vi "MultirunBuilderForNamedLocations2.vi"() -> ()   [LabVIEW 2015]
uses:
  Anemometry Sub Vis/Gen Trav/Spacing.ctl
  Anemometry Sub Vis/Controls/Multi_run_mode.ctl
  MultirunBuilderSubVIs/MRBRowTaskSelector.ctl
  Anemometry Sub Vis/File/Setup_Filetype.ctl
  Anemometry Sub Vis/Controls/Tunnel_Coordinates.ctl
  Anemometry Sub Vis/Globals/Meas_global.vi
  MultirunBuilderSubVIs/MRCMDFBGlobal.vi
  MultirunBuilderSubVIs/Set Speed Only.vi
  MultirunBuilderSubVIs/Wait (minutes).vi
  MultirunBuilderSubVIs/Single Measurement.vi
  MultirunBuilderSubVIs/Auto Calibrate.vi
  MultirunBuilderSubVIs/MoveTT.vi
panel:
  in  "Vert.Z-Locations 2":dbl[](array[numeric])=[12.7, 19.05, 25.4]
  in  "TaskArray":T3(array[cluster])=[{"Start X"=-3390.0, "Start Y"=-113.0, "Start Z"=780.0, "End X"=-3390.0, "End Y"=-113.0, "End Z"=780.0, "No. of pts."=0, "Spacing"=enum."Linear", "Filename"=path "", "Tunnel Speed"=7.64, "Averaging time (min)"=0.0, "Extra Commands"="", "Carrier_1 Q (l/min)"=0.0, "Carrier_2 Q (l/min)"=0.0, "Trace Gas Concentration (%)"=0.0, "Specific Arguments"="", "Comments"="Tunnel Warm Up", "Row No"=0, "Row Type Selector"=enum."Set Tunnel Speed Only", "Completion time"="", "Row Duration (mins)"=10.0, "No. of Valid pts."=0, "Meas Setup File"=""}, {"Start X"=-3390.0, "Start Y"=-113.0, "Start Z"=780.0, "End X"=-3390.0, "End Y"=-113.0, "End Z"=780.0, "No. of pts."=0, "Spacing"=enum."Linear", "Filename"=path "", "Tunnel Speed"=7.64, "Averaging time (min)"=0.0, "Extra Commands"="", "Carrier_1 Q (l/min)"=0.0, "Carrier_2 Q (l/min)"=0.0, "Trace Gas Concentration (%)"=0.0, "Specific Arguments"="10", "Comments"="Tunnel Warm Up", "Row No"=0, "Row Type Selector"=enum."Wait (minutes)", "Completion time"="", "Row Duration (mins)"=0.0, "No. of Valid pts."=0, "Meas Setup File"=""}, {"Start X"=0.0, "Start Y"=0.0, "Start Z"=150.0, "End X"=0.0, "End Y"=0.0, "End Z"=150.0, "No. of pts."=0, "Spacing"=enum."Linear", "Filename"=path "", "Tunnel Speed"=7.64, "Averaging time (min)"=0.0, "Extra Commands"="!Work in Tunnel Coordinates", "Carrier_1 Q (l/min)"=0.0, "Carrier_2 Q (l/min)"=0.0, "Trace Gas Concentration (%)"=0.0, "Specific Arguments"="", "Comments"="", "Row No"=0, "Row Type Selector"=enum."Move Traverse Only", "Completion time"="", "Row Duration (mins)"=0.0, "No. of Valid pts."=0, "Meas Setup File"=""}, {"Start X"=0.0, "Start Y"=0.0, "Start Z"=805.0, "End X"=0.0, "End Y"=0.0, "End Z"=805.0, "No. of pts."=0, "Spacing"=enum."Linear", "Filename"=path "", "Tunnel Speed"=7.64, "Averaging time (min)"=0.0, "Extra Commands"="!Work in Tunnel Coordinates", "Carrier_1 Q (l/min)"=0.0, "Carrier_2 Q (l/min)"=0.0, "Trace Gas Concentration (%)"=0.0, "Specific Arguments"="MoveTT.vi;10", "Comments"="", "Row No"=0, "Row Type Selector"=enum."Run VI Named:", "Completion time"="", "Row Duration (mins)"=0.0, "No. of Valid pts."=0, "Meas Setup File"=""}, {"Start X"=-72.9, "Start Y"=-56.5, "Start Z"=12.7, "End X"=-72.9, "End Y"=-56.5, "End Z"=25.4, "No. of pts."=3, "Spacing"=enum."Specified", "Filename"=path "M:/\\Projects\\8773\\Results\\Tunnel1\\AnemometerSurvey.xls", "Tunnel Speed"=7.64, "Averaging time (min)"=1.0, "Extra Commands"="", "Carrier_1 Q (l/min)"=0.0, "Carrier_2 Q (l/min)"=0.0, "Trace Gas Concentration (%)"=0.0, "Specific Arguments"="Z= ;12.7;19.1;25.4\r", "Comments"="Anemo1", "Row No"=0, "Row Type Selector"=enum."Vertical Profile", "Completion time"="", "Row Duration (mins)"=0.0, "No. of Valid pts."=0, "Meas Setup File"="Current_Setup.xls"}, {"Start X"=-458.4, "Start Y"=87.9, "Start Z"=25.6, "End X"=-458.4, "End Y"=87.9, "End Z"=38.3, "No. of pts."=3, "Spacing"=enum."Specified", "Filename"=path "M:/\\Projects\\8773\\Results\\Tunnel1\\AnemometerSurvey.xls", "Tunnel Speed"=7.64, "Averaging time (min)"=1.0, "Extra Commands"="", "Carrier_1 Q (l/min)"=0.0, "Carrier_2 Q (l/min)"=0.0, "Trace Gas Concentration (%)"=0.0, "Specific Arguments"="Z= ;25.6;32.0;38.3\r", "Comments"="Anemo2", "Row No"=0, "Row Type Selector"=enum."Vertical Profile", "Completion time"="", "Row Duration (mins)"=0.0, "No. of Valid pts."=0, "Meas Setup File"="Current_Setup.xls"}, {"Start X"=0.0, "Start Y"=0.0, "Start Z"=150.0, "End X"=0.0, "End Y"=0.0, "End Z"=150.0, "No. of pts."=0, "Spacing"=enum."Linear", "Filename"=path "", "Tunnel Speed"=7.64, "Averaging time (min)"=0.0, "Extra Commands"="!Work in Tunnel Coordinates", "Carrier_1 Q (l/min)"=0.0, "Carrier_2 Q (l/min)"=0.0, "Trace Gas Concentration (%)"=0.0, "Specific Arguments"="", "Comments"="", "Row No"=0, "Row Type Selector"=enum."Move Traverse Only", "Completion time"="", "Row Duration (mins)"=0.0, "No. of Valid pts."=0, "Meas Setup File"=""}, {"Start X"=0.0, "Start Y"=0.0, "Start Z"=805.0, "End X"=0.0, "End Y"=0.0, "End Z"=805.0, "No. of pts."=0, "Spacing"=enum."Linear", "Filename"=path "", "Tunnel Speed"=7.64, "Averaging time (min)"=0.0, "Extra Commands"="!Work in Tunnel Coordinates", "Carrier_1 Q (l/min)"=0.0, "Carrier_2 Q (l/min)"=0.0, "Trace Gas Concentration (%)"=0.0, "Specific Arguments"="MoveTT.vi;30", "Comments"="", "Row No"=0, "Row Type Selector"=enum."Run VI Named:", "Completion time"="", "Row Duration (mins)"=0.0, "No. of Valid pts."=0, "Meas Setup File"=""}, {"Start X"=-72.9, "Start Y"=-56.5, "Start Z"=12.7, "End X"=-72.9, "End Y"=-56.5, "End Z"=25.4, "No. of pts."=3, "Spacing"=enum."Specified", "Filename"=path "M:/\\Projects\\8773\\Results\\Tunnel1\\AnemometerSurvey.xls", "Tunnel Speed"=7.64, "Averaging time (min)"=1.0, "Extra Commands"="", "Carrier_1 Q (l/min)"=0.0, "Carrier_2 Q (l/min)"=0.0, "Trace Gas Concentration (%)"=0.0, "Specific Arguments"="Z= ;12.7;19.1;25.4\r", "Comments"="Anemo1", "Row No"=0, "Row Type Selector"=enum."Vertical Profile", "Completion time"="", "Row Duration (mins)"=0.0, "No. of Valid pts."=0, "Meas Setup File"="Current_Setup.xls"}, {"Start X"=-458.4, "Start Y"=87.9, "Start Z"=25.6, "End X"=-458.4, "End Y"=87.9, "End Z"=38.3, "No. of pts."=3, "Spacing"=enum."Specified", "Filename"=path "M:/\\Projects\\8773\\Results\\Tunnel1\\AnemometerSurvey.xls", "Tunnel Speed"=7.64, "Averaging time (min)"=1.0, "Extra Commands"="", "Carrier_1 Q (l/min)"=0.0, "Carrier_2 Q (l/min)"=0.0, "Trace Gas Concentration (%)"=0.0, "Specific Arguments"="Z= ;25.6;32.0;38.3\r", "Comments"="Anemo2", "Row No"=0, "Row Type Selector"=enum."Vertical Profile", "Completion time"="", "Row Duration (mins)"=0.0, "No. of Valid pts."=0, "Meas Setup File"="Current_Setup.xls"}, {"Start X"=0.0, "Start Y"=0.0, "Start Z"=150.0, "End X"=0.0, "End Y"=0.0, "End Z"=150.0, "No. of pts."=0, "Spacing"=enum."Linear", "Filename"=path "", "Tunnel Speed"=7.64, "Averaging time (min)"=0.0, "Extra Commands"="!Work in Tunnel Coordinates", "Carrier_1 Q (l/min)"=0.0, "Carrier_2 Q (l/min)"=0.0, "Trace Gas Concentration (%)"=0.0, "Specific Arguments"="", "Comments"="", "Row No"=0, "Row Type Selector"=enum."Move Traverse Only", "Completion time"="", "Row Duration (mins)"=0.0, "No. of Valid pts."=0, "Meas Setup File"=""}, {"Start X"=0.0, "Start Y"=0.0, "Start Z"=805.0, "End X"=0.0, "End Y"=0.0, "End Z"=805.0, "No. of pts."=0, "Spacing"=enum."Linear", "Filename"=path "", "Tunnel Speed"=7.64, "Averaging time (min)"=0.0, "Extra Commands"="!Work in Tunnel Coordinates", "Carrier_1 Q (l/min)"=0.0, "Carrier_2 Q (l/min)"=0.0, "Trace Gas Concentration (%)"=0.0, "Specific Arguments"="MoveTT.vi;50", "Comments"="", "Row No"=0, "Row Type Selector"=enum."Run VI Named:", "Completion time"="", "Row Duration (mins)"=0.0, "No. of Valid pts."=0, "Meas Setup File"=""}, {"Start X"=-72.9, "Start Y"=-56.5, "Start Z"=12.7, "End X"=-72.9, "End Y"=-56.5, "End Z"=25.4, "No. of pts."=3, "Spacing"=enum."Specified", "Filename"=path "M:/\\Projects\\8773\\Results\\Tunnel1\\AnemometerSurvey.xls", "Tunnel Speed"=7.64, "Averaging time (min)"=1.0, "Extra Commands"="", "Carrier_1 Q (l/min)"=0.0, "Carrier_2 Q (l/min)"=0.0, "Trace Gas Concentration (%)"=0.0, "Specific Arguments"="Z= ;12.7;19.1;25.4\r", "Comments"="Anemo1", "Row No"=0, "Row Type Selector"=enum."Vertical Profile", "Completion time"="", "Row Duration (mins)"=0.0, "No. of Valid pts."=0, "Meas Setup File"="Current_Setup.xls"}, {"Start X"=-458.4, "Start Y"=87.9, "Start Z"=25.6, "End X"=-458.4, "End Y"=87.9, "End Z"=38.3, "No. of pts."=3, "Spacing"=enum."Specified", "Filename"=path "M:/\\Projects\\8773\\Results\\Tunnel1\\AnemometerSurvey.xls", "Tunnel Speed"=7.64, "Averaging time (min)"=1.0, "Extra Commands"="", "Carrier_1 Q (l/min)"=0.0, "Carrier_2 Q (l/min)"=0.0, "Trace Gas Concentration (%)"=0.0, "Specific Arguments"="Z= ;25.6;32.0;38.3\r", "Comments"="Anemo2", "Row No"=0, "Row Type Selector"=enum."Vertical Profile", "Completion time"="", "Row Duration (mins)"=0.0, "No. of Valid pts."=0, "Meas Setup File"="Current_Setup.xls"}, {"Start X"=0.0, "Start Y"=0.0, "Start Z"=150.0, "End X"=0.0, "End Y"=0.0, "End Z"=150.0, "No. of pts."=0, "Spacing"=enum."Linear", "Filename"=path "", "Tunnel Speed"=7.64, "Averaging time (min)"=0.0, "Extra Commands"="!Work in Tunnel Coordinates", "Carrier_1 Q (l/min)"=0.0, "Carrier_2 Q (l/min)"=0.0, "Trace Gas Concentration (%)"=0.0, "Specific Arguments"="", "Comments"="", "Row No"=0, "Row Type Selector"=enum."Move Traverse Only", "Completion time"="", "Row Duration (mins)"=0.0, "No. of Valid pts."=0, "Meas Setup File"=""}, {"Start X"=0.0, "Start Y"=0.0, "Start Z"=805.0, "End X"=0.0, "End Y"=0.0, "End Z"=805.0, "No. of pts."=0, "Spacing"=enum."Linear", "Filename"=path "", "Tunnel Speed"=7.64, "Averaging time (min)"=0.0, "Extra Commands"="!Work in Tunnel Coordinates", "Carrier_1 Q (l/min)"=0.0, "Carrier_2 Q (l/min)"=0.0, "Trace Gas Concentration (%)"=0.0, "Specific Arguments"="MoveTT.vi;70", "Comments"="", "Row No"=0, "Row Type Selector"=enum."Run VI Named:", "Completion time"="", "Row Duration (mins)"=0.0, "No. of Valid pts."=0, "Meas Setup File"=""}, {"Start X"=-72.9, "Start Y"=-56.5, "Start Z"=12.7, "End X"=-72.9, "End Y"=-56.5, "End Z"=25.4, "No. of pts."=3, "Spacing"=enum."Specified", "Filename"=path "M:/\\Projects\\8773\\Results\\Tunnel1\\AnemometerSurvey.xls", "Tunnel Speed"=7.64, "Averaging time (min)"=1.0, "Extra Commands"="", "Carrier_1 Q (l/min)"=0.0, "Carrier_2 Q (l/min)"=0.0, "Trace Gas Concentration (%)"=0.0, "Specific Arguments"="Z= ;12.7;19.1;25.4\r", "Comments"="Anemo1", "Row No"=0, "Row Type Selector"=enum."Vertical Profile", "Completion time"="", "Row Duration (mins)"=0.0, "No. of Valid pts."=0, "Meas Setup File"="Current_Setup.xls"}, {"Start X"=-458.4, "Start Y"=87.9, "Start Z"=25.6, "End X"=-458.4, "End Y"=87.9, "End Z"=38.3, "No. of pts."=3, "Spacing"=enum."Specified", "Filename"=path "M:/\\Projects\\8773\\Results\\Tunnel1\\AnemometerSurvey.xls", "Tunnel Speed"=7.64, "Averaging time (min)"=1.0, "Extra Commands"="", "Carrier_1 Q (l/min)"=0.0, "Carrier_2 Q (l/min)"=0.0, "Trace Gas Concentration (%)"=0.0, "Specific Arguments"="Z= ;25.6;32.0;38.3\r", "Comments"="Anemo2", "Row No"=0, "Row Type Selector"=enum."Vertical Profile", "Completion time"="", "Row Duration (mins)"=0.0, "No. of Valid pts."=0, "Meas Setup File"="Current_Setup.xls"}, {"Start X"=0.0, "Start Y"=0.0, "Start Z"=150.0, "End X"=0.0, "End Y"=0.0, "End Z"=150.0, "No. of pts."=0, "Spacing"=enum."Linear", "Filename"=path "", "Tunnel Speed"=7.64, "Averaging time (min)"=0.0, "Extra Commands"="!Work in Tunnel Coordinates", "Carrier_1 Q (l/min)"=0.0, "Carrier_2 Q (l/min)"=0.0, "Trace Gas Concentration (%)"=0.0, "Specific Arguments"="", "Comments"="", "Row No"=0, "Row Type Selector"=enum."Move Traverse Only", "Completion time"="", "Row Duration (mins)"=0.0, "No. of Valid pts."=0, "Meas Setup File"=""}, {"Start X"=0.0, "Start Y"=0.0, "Start Z"=805.0, "End X"=0.0, "End Y"=0.0, "End Z"=805.0, "No. of pts."=0, "Spacing"=enum."Linear", "Filename"=path "", "Tunnel Speed"=7.64, "Averaging time (min)"=0.0, "Extra Commands"="!Work in Tunnel Coordinates", "Carrier_1 Q (l/min)"=0.0, "Carrier_2 Q (l/min)"=0.0, "Trace Gas Concentration (%)"=0.0, "Specific Arguments"="MoveTT.vi;90", "Comments"="", "Row No"=0, "Row Type Selector"=enum."Run VI Named:", "Completion time"="", "Row Duration (mins)"=0.0, "No. of Valid pts."=0, "Meas Setup File"=""}, {"Start X"=-72.9, "Start Y"=-56.5, "Start Z"=12.7, "End X"=-72.9, "End Y"=-56.5, "End Z"=25.4, "No. of pts."=3, "Spacing"=enum."Specified", "Filename"=path "M:/\\Projects\\8773\\Results\\Tunnel1\\AnemometerSurvey.xls", "Tunnel Speed"=7.64, "Averaging time (min)"=1.0, "Extra Commands"="", "Carrier_1 Q (l/min)"=0.0, "Carrier_2 Q (l/min)"=0.0, "Trace Gas Concentration (%)"=0.0, "Specific Arguments"="Z= ;12.7;19.1;25.4\r", "Comments"="Anemo1", "Row No"=0, "Row Type Selector"=enum."Vertical Profile", "Completion time"="", "Row Duration (mins)"=0.0, "No. of Valid pts."=0, "Meas Setup File"="Current_Setup.xls"}, {"Start X"=-458.4, "Start Y"=87.9, "Start Z"=25.6, "End X"=-458.4, "End Y"=87.9, "End Z"=38.3, "No. of pts."=3, "Spacing"=enum."Specified", "Filename"=path "M:/\\Projects\\8773\\Results\\Tunnel1\\AnemometerSurvey.xls", "Tunnel Speed"=7.64, "Averaging time (min)"=1.0, "Extra Commands"="", "Carrier_1 Q (l/min)"=0.0, "Carrier_2 Q (l/min)"=0.0, "Trace Gas Concentration (%)"=0.0, "Specific Arguments"="Z= ;25.6;32.0;38.3\r", "Comments"="Anemo2", "Row No"=0, "Row Type Selector"=enum."Vertical Profile", "Completion time"="", "Row Duration (mins)"=0.0, "No. of Valid pts."=0, "Meas Setup File"="Current_Setup.xls"}, {"Start X"=0.0, "Start Y"=0.0, "Start Z"=150.0, "End X"=0.0, "End Y"=0.0, "End Z"=150.0, "No. of pts."=0, "Spacing"=enum."Linear", "Filename"=path "", "Tunnel Speed"=7.64, "Averaging time (min)"=0.0, "Extra Commands"="!Work in Tunnel Coordinates", "Carrier_1 Q (l/min)"=0.0, "Carrier_2 Q (l/min)"=0.0, "Trace Gas Concentration (%)"=0.0, "Specific Arguments"="", "Comments"="", "Row No"=0, "Row Type Selector"=enum."Move Traverse Only", "Completion time"="", "Row Duration (mins)"=0.0, "No. of Valid pts."=0, "Meas Setup File"=""}, {"Start X"=0.0, "Start Y"=0.0, "Start Z"=805.0, "End X"=0.0, "End Y"=0.0, "End Z"=805.0, "No. of pts."=0, "Spacing"=enum."Linear", "Filename"=path "", "Tunnel Speed"=7.64, "Averaging time (min)"=0.0, "Extra Commands"="!Work in Tunnel Coordinates", "Carrier_1 Q (l/min)"=0.0, "Carrier_2 Q (l/min)"=0.0, "Trace Gas Concentration (%)"=0.0, "Specific Arguments"="MoveTT.vi;110", "Comments"="", "Row No"=0, "Row Type Selector"=enum."Run VI Named:", "Completion time"="", "Row Duration (mins)"=0.0, "No. of Valid pts."=0, "Meas Setup File"=""}, {"Start X"=-72.9, "Start Y"=-56.5, "Start Z"=12.7, "End X"=-72.9, "End Y"=-56.5, "End Z"=25.4, "No. of pts."=3, "Spacing"=enum."Specified", "Filename"=path "M:/\\Projects\\8773\\Results\\Tunnel1\\AnemometerSurvey.xls", "Tunnel Speed"=7.64, "Averaging time (min)"=1.0, "Extra Commands"="", "Carrier_1 Q (l/min)"=0.0, "Carrier_2 Q (l/min)"=0.0, "Trace Gas Concentration (%)"=0.0, "Specific Arguments"="Z= ;12.7;19.1;25.4\r", "Comments"="Anemo1", "Row No"=0, "Row Type Selector"=enum."Vertical Profile", "Completion time"="", "Row Duration (mins)"=0.0, "No. of Valid pts."=0, "Meas Setup File"="Current_Setup.xls"}, {"Start X"=-458.4, "Start Y"=87.9, "Start Z"=25.6, "End X"=-458.4, "End Y"=87.9, "End Z"=38.3, "No. of pts."=3, "Spacing"=enum."Specified", "Filename"=path "M:/\\Projects\\8773\\Results\\Tunnel1\\AnemometerSurvey.xls", "Tunnel Speed"=7.64, "Averaging time (min)"=1.0, "Extra Commands"="", "Carrier_1 Q (l/min)"=0.0, "Carrier_2 Q (l/min)"=0.0, "Trace Gas Concentration (%)"=0.0, "Specific Arguments"="Z= ;25.6;32.0;38.3\r", "Comments"="Anemo2", "Row No"=0, "Row Type Selector"=enum."Vertical Profile", "Completion time"="", "Row Duration (mins)"=0.0, "No. of Valid pts."=0, "Meas Setup File"="Current_Setup.xls"}, {"Start X"=0.0, "Start Y"=0.0, "Start Z"=150.0, "End X"=0.0, "End Y"=0.0, "End Z"=150.0, "No. of pts."=0, "Spacing"=enum."Linear", "Filename"=path "", "Tunnel Speed"=7.64, "Averaging time (min)"=0.0, "Extra Commands"="!Work in Tunnel Coordinates", "Carrier_1 Q (l/min)"=0.0, "Carrier_2 Q (l/min)"=0.0, "Trace Gas Concentration (%)"=0.0, "Specific Arguments"="", "Comments"="", "Row No"=0, "Row Type Selector"=enum."Move Traverse Only", "Completion time"="", "Row Duration (mins)"=0.0, "No. of Valid pts."=0, "Meas Setup File"=""}, {"Start X"=0.0, "Start Y"=0.0, "Start Z"=805.0, "End X"=0.0, "End Y"=0.0, "End Z"=805.0, "No. of pts."=0, "Spacing"=enum."Linear", "Filename"=path "", "Tunnel Speed"=7.64, "Averaging time (min)"=0.0, "Extra Commands"="!Work in Tunnel Coordinates", "Carrier_1 Q (l/min)"=0.0, "Carrier_2 Q (l/min)"=0.0, "Trace Gas Concentration (%)"=0.0, "Specific Arguments"="MoveTT.vi;130", "Comments"="", "Row No"=0, "Row Type Selector"=enum."Run VI Named:", "Completion time"="", "Row Duration (mins)"=0.0, "No. of Valid pts."=0, "Meas Setup File"=""}, {"Start X"=-72.9, "Start Y"=-56.5, "Start Z"=12.7, "End X"=-72.9, "End Y"=-56.5, "End Z"=25.4, "No. of pts."=3, "Spacing"=enum."Specified", "Filename"=path "M:/\\Projects\\8773\\Results\\Tunnel1\\AnemometerSurvey.xls", "Tunnel Speed"=7.64, "Averaging time (min)"=1.0, "Extra Commands"="", "Carrier_1 Q (l/min)"=0.0, "Carrier_2 Q (l/min)"=0.0, "Trace Gas Concentration (%)"=0.0, "Specific Arguments"="Z= ;12.7;19.1;25.4\r", "Comments"="Anemo1", "Row No"=0, "Row Type Selector"=enum."Vertical Profile", "Completion time"="", "Row Duration (mins)"=0.0, "No. of Valid pts."=0, "Meas Setup File"="Current_Setup.xls"}, {"Start X"=-458.4, "Start Y"=87.9, "Start Z"=25.6, "End X"=-458.4, "End Y"=87.9, "End Z"=38.3, "No. of pts."=3, "Spacing"=enum."Specified", "Filename"=path "M:/\\Projects\\8773\\Results\\Tunnel1\\AnemometerSurvey.xls", "Tunnel Speed"=7.64, "Averaging time (min)"=1.0, "Extra Commands"="", "Carrier_1 Q (l/min)"=0.0, "Carrier_2 Q (l/min)"=0.0, "Trace Gas Concentration (%)"=0.0, "Specific Arguments"="Z= ;25.6;32.0;38.3\r", "Comments"="Anemo2", "Row No"=0, "Row Type Selector"=enum."Vertical Profile", "Completion time"="", "Row Duration (mins)"=0.0, "No. of Valid pts."=0, "Meas Setup File"="Current_Setup.xls"}, {"Start X"=0.0, "Start Y"=0.0, "Start Z"=150.0, "End X"=0.0, "End Y"=0.0, "End Z"=150.0, "No. of pts."=0, "Spacing"=enum."Linear", "Filename"=path "", "Tunnel Speed"=7.64, "Averaging time (min)"=0.0, "Extra Commands"="!Work in Tunnel Coordinates", "Carrier_1 Q (l/min)"=0.0, "Carrier_2 Q (l/min)"=0.0, "Trace Gas Concentration (%)"=0.0, "Specific Arguments"="", "Comments"="", "Row No"=0, "Row Type Selector"=enum."Move Traverse Only", "Completion time"="", "Row Duration (mins)"=0.0, "No. of Valid pts."=0, "Meas Setup File"=""}, {"Start X"=0.0, "Start Y"=0.0, "Start Z"=805.0, "End X"=0.0, "End Y"=0.0, "End Z"=805.0, "No. of pts."=0, "Spacing"=enum."Linear", "Filename"=path "", "Tunnel Speed"=7.64, "Averaging time (min)"=0.0, "Extra Commands"="!Work in Tunnel Coordinates", "Carrier_1 Q (l/min)"=0.0, "Carrier_2 Q (l/min)"=0.0, "Trace Gas Concentration (%)"=0.0, "Specific Arguments"="MoveTT.vi;150", "Comments"="", "Row No"=0, "Row Type Selector"=enum."Run VI Named:", "Completion time"="", "Row Duration (mins)"=0.0, "No. of Valid pts."=0, "Meas Setup File"=""}, {"Start X"=-72.9, "Start Y"=-56.5, "Start Z"=12.7, "End X"=-72.9, "End Y"=-56.5, "End Z"=25.4, "No. of pts."=3, "Spacing"=enum."Specified", "Filename"=path "M:/\\Projects\\8773\\Results\\Tunnel1\\AnemometerSurvey.xls", "Tunnel Speed"=7.64, "Averaging time (min)"=1.0, "Extra Commands"="", "Carrier_1 Q (l/min)"=0.0, "Carrier_2 Q (l/min)"=0.0, "Trace Gas Concentration (%)"=0.0, "Specific Arguments"="Z= ;12.7;19.1;25.4\r", "Comments"="Anemo1", "Row No"=0, "Row Type Selector"=enum."Vertical Profile", "Completion time"="", "Row Duration (mins)"=0.0, "No. of Valid pts."=0, "Meas Setup File"="Current_Setup.xls"}, {"Start X"=-458.4, "Start Y"=87.9, "Start Z"=25.6, "End X"=-458.4, "End Y"=87.9, "End Z"=38.3, "No. of pts."=3, "Spacing"=enum."Specified", "Filename"=path "M:/\\Projects\\8773\\Results\\Tunnel1\\AnemometerSurvey.xls", "Tunnel Speed"=7.64, "Averaging time (min)"=1.0, "Extra Commands"="", "Carrier_1 Q (l/min)"=0.0, "Carrier_2 Q (l/min)"=0.0, "Trace Gas Concentration (%)"=0.0, "Specific Arguments"="Z= ;25.6;32.0;38.3\r", "Comments"="Anemo2", "Row No"=0, "Row Type Selector"=enum."Vertical Profile", "Completion time"="", "Row Duration (mins)"=0.0, "No. of Valid pts."=0, "Meas Setup File"="Current_Setup.xls"}, {"Start X"=0.0, "Start Y"=0.0, "Start Z"=150.0, "End X"=0.0, "End Y"=0.0, "End Z"=150.0, "No. of pts."=0, "Spacing"=enum."Linear", "Filename"=path "", "Tunnel Speed"=7.64, "Averaging time (min)"=0.0, "Extra Commands"="!Work in Tunnel Coordinates", "Carrier_1 Q (l/min)"=0.0, "Carrier_2 Q (l/min)"=0.0, "Trace Gas Concentration (%)"=0.0, "Specific Arguments"="", "Comments"="", "Row No"=0, "Row Type Selector"=enum."Move Traverse Only", "Completion time"="", "Row Duration (mins)"=0.0, "No. of Valid pts."=0, "Meas Setup File"=""}, {"Start X"=0.0, "Start Y"=0.0, "Start Z"=805.0, "End X"=0.0, "End Y"=0.0, "End Z"=805.0, "No. of pts."=0, "Spacing"=enum."Linear", "Filename"=path "", "Tunnel Speed"=7.64, "Averaging time (min)"=0.0, "Extra Commands"="!Work in Tunnel Coordinates", "Carrier_1 Q (l/min)"=0.0, "Carrier_2 Q (l/min)"=0.0, "Trace Gas Concentration (%)"=0.0, "Specific Arguments"="MoveTT.vi;170", "Comments"="", "Row No"=0, "Row Type Selector"=enum."Run VI Named:", "Completion time"="", "Row Duration (mins)"=0.0, "No. of Valid pts."=0, "Meas Setup File"=""}, {"Start X"=-72.9, "Start Y"=-56.5, "Start Z"=12.7, "End X"=-72.9, "End Y"=-56.5, "End Z"=25.4, "No. of pts."=3, "Spacing"=enum."Specified", "Filename"=path "M:/\\Projects\\8773\\Results\\Tunnel1\\AnemometerSurvey.xls", "Tunnel Speed"=7.64, "Averaging time (min)"=1.0, "Extra Commands"="", "Carrier_1 Q (l/min)"=0.0, "Carrier_2 Q (l/min)"=0.0, "Trace Gas Concentration (%)"=0.0, "Specific Arguments"="Z= ;12.7;19.1;25.4\r", "Comments"="Anemo1", "Row No"=0, "Row Type Selector"=enum."Vertical Profile", "Completion time"="", "Row Duration (mins)"=0.0, "No. of Valid pts."=0, "Meas Setup File"="Current_Setup.xls"}, {"Start X"=-458.4, "Start Y"=87.9, "Start Z"=25.6, "End X"=-458.4, "End Y"=87.9, "End Z"=38.3, "No. of pts."=3, "Spacing"=enum."Specified", "Filename"=path "M:/\\Projects\\8773\\Results\\Tunnel1\\AnemometerSurvey.xls", "Tunnel Speed"=7.64, "Averaging time (min)"=1.0, "Extra Commands"="", "Carrier_1 Q (l/min)"=0.0, "Carrier_2 Q (l/min)"=0.0, "Trace Gas Concentration (%)"=0.0, "Specific Arguments"="Z= ;25.6;32.0;38.3\r", "Comments"="Anemo2", "Row No"=0, "Row Type Selector"=enum."Vertical Profile", "Completion time"="", "Row Duration (mins)"=0.0, "No. of Valid pts."=0, "Meas Setup File"="Current_Setup.xls"}, {"Start X"=0.0, "Start Y"=0.0, "Start Z"=150.0, "End X"=0.0, "End Y"=0.0, "End Z"=150.0, "No. of pts."=0, "Spacing"=enum."Linear", "Filename"=path "", "Tunnel Speed"=7.64, "Averaging time (min)"=0.0, "Extra Commands"="!Work in Tunnel Coordinates", "Carrier_1 Q (l/min)"=0.0, "Carrier_2 Q (l/min)"=0.0, "Trace Gas Concentration (%)"=0.0, "Specific Arguments"="", "Comments"="", "Row No"=0, "Row Type Selector"=enum."Move Traverse Only", "Completion time"="", "Row Duration (mins)"=0.0, "No. of Valid pts."=0, "Meas Setup File"=""}, {"Start X"=0.0, "Start Y"=0.0, "Start Z"=805.0, "End X"=0.0, "End Y"=0.0, "End Z"=805.0, "No. of pts."=0, "Spacing"=enum."Linear", "Filename"=path "", "Tunnel Speed"=7.64, "Averaging time (min)"=0.0, "Extra Commands"="!Work in Tunnel Coordinates", "Carrier_1 Q (l/min)"=0.0, "Carrier_2 Q (l/min)"=0.0, "Trace Gas Concentration (%)"=0.0, "Specific Arguments"="MoveTT.vi;190", "Comments"="", "Row No"=0, "Row Type Selector"=enum."Run VI Named:", "Completion time"="", "Row Duration (mins)"=0.0, "No. of Valid pts."=0, "Meas Setup File"=""}, {"Start X"=-72.9, "Start Y"=-56.5, "Start Z"=12.7, "End X"=-72.9, "End Y"=-56.5, "End Z"=25.4, "No. of pts."=3, "Spacing"=enum."Specified", "Filename"=path "M:/\\Projects\\8773\\Results\\Tunnel1\\AnemometerSurvey.xls", "Tunnel Speed"=7.64, "Averaging time (min)"=1.0, "Extra Commands"="", "Carrier_1 Q (l/min)"=0.0, "Carrier_2 Q (l/min)"=0.0, "Trace Gas Concentration (%)"=0.0, "Specific Arguments"="Z= ;12.7;19.1;25.4\r", "Comments"="Anemo1", "Row No"=0, "Row Type Selector"=enum."Vertical Profile", "Completion time"="", "Row Duration (mins)"=0.0, "No. of Valid pts."=0, "Meas Setup File"="Current_Setup.xls"}, {"Start X"=-458.4, "Start Y"=87.9, "Start Z"=25.6, "End X"=-458.4, "End Y"=87.9, "End Z"=38.3, "No. of pts."=3, "Spacing"=enum."Specified", "Filename"=path "M:/\\Projects\\8773\\Results\\Tunnel1\\AnemometerSurvey.xls", "Tunnel Speed"=7.64, "Averaging time (min)"=1.0, "Extra Commands"="", "Carrier_1 Q (l/min)"=0.0, "Carrier_2 Q (l/min)"=0.0, "Trace Gas Concentration (%)"=0.0, "Specific Arguments"="Z= ;25.6;32.0;38.3\r", "Comments"="Anemo2", "Row No"=0, "Row Type Selector"=enum."Vertical Profile", "Completion time"="", "Row Duration (mins)"=0.0, "No. of Valid pts."=0, "Meas Setup File"="Current_Setup.xls"}, {"Start X"=0.0, "Start Y"=0.0, "Start Z"=150.0, "End X"=0.0, "End Y"=0.0, "End Z"=150.0, "No. of pts."=0, "Spacing"=enum."Linear", "Filename"=path "", "Tunnel Speed"=7.64, "Averaging time (min)"=0.0, "Extra Commands"="!Work in Tunnel Coordinates", "Carrier_1 Q (l/min)"=0.0, "Carrier_2 Q (l/min)"=0.0, "Trace Gas Concentration (%)"=0.0, "Specific Arguments"="", "Comments"="", "Row No"=0, "Row Type Selector"=enum."Move Traverse Only", "Completion time"="", "Row Duration (mins)"=0.0, "No. of Valid pts."=0, "Meas Setup File"=""}, {"Start X"=0.0, "Start Y"=0.0, "Start Z"=805.0, "End X"=0.0, "End Y"=0.0, "End Z"=805.0, "No. of pts."=0, "Spacing"=enum."Linear", "Filename"=path "", "Tunnel Speed"=7.64, "Averaging time (min)"=0.0, "Extra Commands"="!Work in Tunnel Coordinates", "Carrier_1 Q (l/min)"=0.0, "Carrier_2 Q (l/min)"=0.0, "Trace Gas Concentration (%)"=0.0, "Specific Arguments"="MoveTT.vi;210", "Comments"="", "Row No"=0, "Row Type Selector"=enum."Run VI Named:", "Completion time"="", "Row Duration (mins)"=0.0, "No. of Valid pts."=0, "Meas Setup File"=""}, {"Start X"=-72.9, "Start Y"=-56.5, "Start Z"=12.7, "End X"=-72.9, "End Y"=-56.5, "End Z"=25.4, "No. of pts."=3, "Spacing"=enum."Specified", "Filename"=path "M:/\\Projects\\8773\\Results\\Tunnel1\\AnemometerSurvey.xls", "Tunnel Speed"=7.64, "Averaging time (min)"=1.0, "Extra Commands"="", "Carrier_1 Q (l/min)"=0.0, "Carrier_2 Q (l/min)"=0.0, "Trace Gas Concentration (%)"=0.0, "Specific Arguments"="Z= ;12.7;19.1;25.4\r", "Comments"="Anemo1", "Row No"=0, "Row Type Selector"=enum."Vertical Profile", "Completion time"="", "Row Duration (mins)"=0.0, "No. of Valid pts."=0, "Meas Setup File"="Current_Setup.xls"}, {"Start X"=-458.4, "Start Y"=87.9, "Start Z"=25.6, "End X"=-458.4, "End Y"=87.9, "End Z"=38.3, "No. of pts."=3, "Spacing"=enum."Specified", "Filename"=path "M:/\\Projects\\8773\\Results\\Tunnel1\\AnemometerSurvey.xls", "Tunnel Speed"=7.64, "Averaging time (min)"=1.0, "Extra Commands"="", "Carrier_1 Q (l/min)"=0.0, "Carrier_2 Q (l/min)"=0.0, "Trace Gas Concentration (%)"=0.0, "Specific Arguments"="Z= ;25.6;32.0;38.3\r", "Comments"="Anemo2", "Row No"=0, "Row Type Selector"=enum."Vertical Profile", "Completion time"="", "Row Duration (mins)"=0.0, "No. of Valid pts."=0, "Meas Setup File"="Current_Setup.xls"}, {"Start X"=0.0, "Start Y"=0.0, "Start Z"=150.0, "End X"=0.0, "End Y"=0.0, "End Z"=150.0, "No. of pts."=0, "Spacing"=enum."Linear", "Filename"=path "", "Tunnel Speed"=7.64, "Averaging time (min)"=0.0, "Extra Commands"="!Work in Tunnel Coordinates", "Carrier_1 Q (l/min)"=0.0, "Carrier_2 Q (l/min)"=0.0, "Trace Gas Concentration (%)"=0.0, "Specific Arguments"="", "Comments"="", "Row No"=0, "Row Type Selector"=enum."Move Traverse Only", "Completion time"="", "Row Duration (mins)"=0.0, "No. of Valid pts."=0, "Meas Setup File"=""}, {"Start X"=0.0, "Start Y"=0.0, "Start Z"=805.0, "End X"=0.0, "End Y"=0.0, "End Z"=805.0, "No. of pts."=0, "Spacing"=enum."Linear", "Filename"=path "", "Tunnel Speed"=7.64, "Averaging time (min)"=0.0, "Extra Commands"="!Work in Tunnel Coordinates", "Carrier_1 Q (l/min)"=0.0, "Carrier_2 Q (l/min)"=0.0, "Trace Gas Concentration (%)"=0.0, "Specific Arguments"="MoveTT.vi;230", "Comments"="", "Row No"=0, "Row Type Selector"=enum."Run VI Named:", "Completion time"="", "Row Duration (mins)"=0.0, "No. of Valid pts."=0, "Meas Setup File"=""}, {"Start X"=-72.9, "Start Y"=-56.5, "Start Z"=12.7, "End X"=-72.9, "End Y"=-56.5, "End Z"=25.4, "No. of pts."=3, "Spacing"=enum."Specified", "Filename"=path "M:/\\Projects\\8773\\Results\\Tunnel1\\AnemometerSurvey.xls", "Tunnel Speed"=7.64, "Averaging time (min)"=1.0, "Extra Commands"="", "Carrier_1 Q (l/min)"=0.0, "Carrier_2 Q (l/min)"=0.0, "Trace Gas Concentration (%)"=0.0, "Specific Arguments"="Z= ;12.7;19.1;25.4\r", "Comments"="Anemo1", "Row No"=0, "Row Type Selector"=enum."Vertical Profile", "Completion time"="", "Row Duration (mins)"=0.0, "No. of Valid pts."=0, "Meas Setup File"="Current_Setup.xls"}, {"Start X"=-458.4, "Start Y"=87.9, "Start Z"=25.6, "End X"=-458.4, "End Y"=87.9, "End Z"=38.3, "No. of pts."=3, "Spacing"=enum."Specified", "Filename"=path "M:/\\Projects\\8773\\Results\\Tunnel1\\AnemometerSurvey.xls", "Tunnel Speed"=7.64, "Averaging time (min)"=1.0, "Extra Commands"="", "Carrier_1 Q (l/min)"=0.0, "Carrier_2 Q (l/min)"=0.0, "Trace Gas Concentration (%)"=0.0, "Specific Arguments"="Z= ;25.6;32.0;38.3\r", "Comments"="Anemo2", "Row No"=0, "Row Type Selector"=enum."Vertical Profile", "Completion time"="", "Row Duration (mins)"=0.0, "No. of Valid pts."=0, "Meas Setup File"="Current_Setup.xls"}, {"Start X"=0.0, "Start Y"=0.0, "Start Z"=150.0, "End X"=0.0, "End Y"=0.0, "End Z"=150.0, "No. of pts."=0, "Spacing"=enum."Linear", "Filename"=path "", "Tunnel Speed"=7.64, "Averaging time (min)"=0.0, "Extra Commands"="!Work in Tunnel Coordinates", "Carrier_1 Q (l/min)"=0.0, "Carrier_2 Q (l/min)"=0.0, "Trace Gas Concentration (%)"=0.0, "Specific Arguments"="", "Comments"="", "Row No"=0, "Row Type Selector"=enum."Move Traverse Only", "Completion time"="", "Row Duration (mins)"=0.0, "No. of Valid pts."=0, "Meas Setup File"=""}, {"Start X"=0.0, "Start Y"=0.0, "Start Z"=805.0, "End X"=0.0, "End Y"=0.0, "End Z"=805.0, "No. of pts."=0, "Spacing"=enum."Linear", "Filename"=path "", "Tunnel Speed"=7.64, "Averaging time (min)"=0.0, "Extra Commands"="!Work in Tunnel Coordinates", "Carrier_1 Q (l/min)"=0.0, "Carrier_2 Q (l/min)"=0.0, "Trace Gas Concentration (%)"=0.0, "Specific Arguments"="MoveTT.vi;250", "Comments"="", "Row No"=0, "Row Type Selector"=enum."Run VI Named:", "Completion time"="", "Row Duration (mins)"=0.0, "No. of Valid pts."=0, "Meas Setup File"=""}, {"Start X"=-72.9, "Start Y"=-56.5, "Start Z"=12.7, "End X"=-72.9, "End Y"=-56.5, "End Z"=25.4, "No. of pts."=3, "Spacing"=enum."Specified", "Filename"=path "M:/\\Projects\\8773\\Results\\Tunnel1\\AnemometerSurvey.xls", "Tunnel Speed"=7.64, "Averaging time (min)"=1.0, "Extra Commands"="", "Carrier_1 Q (l/min)"=0.0, "Carrier_2 Q (l/min)"=0.0, "Trace Gas Concentration (%)"=0.0, "Specific Arguments"="Z= ;12.7;19.1;25.4\r", "Comments"="Anemo1", "Row No"=0, "Row Type Selector"=enum."Vertical Profile", "Completion time"="", "Row Duration (mins)"=0.0, "No. of Valid pts."=0, "Meas Setup File"="Current_Setup.xls"}, {"Start X"=-458.4, "Start Y"=87.9, "Start Z"=25.6, "End X"=-458.4, "End Y"=87.9, "End Z"=38.3, "No. of pts."=3, "Spacing"=enum."Specified", "Filename"=path "M:/\\Projects\\8773\\Results\\Tunnel1\\AnemometerSurvey.xls", "Tunnel Speed"=7.64, "Averaging time (min)"=1.0, "Extra Commands"="", "Carrier_1 Q (l/min)"=0.0, "Carrier_2 Q (l/min)"=0.0, "Trace Gas Concentration (%)"=0.0, "Specific Arguments"="Z= ;25.6;32.0;38.3\r", "Comments"="Anemo2", "Row No"=0, "Row Type Selector"=enum."Vertical Profile", "Completion time"="", "Row Duration (mins)"=0.0, "No. of Valid pts."=0, "Meas Setup File"="Current_Setup.xls"}, {"Start X"=0.0, "Start Y"=0.0, "Start Z"=150.0, "End X"=0.0, "End Y"=0.0, "End Z"=150.0, "No. of pts."=0, "Spacing"=enum."Linear", "Filename"=path "", "Tunnel Speed"=7.64, "Averaging time (min)"=0.0, "Extra Commands"="!Work in Tunnel Coordinates", "Carrier_1 Q (l/min)"=0.0, "Carrier_2 Q (l/min)"=0.0, "Trace Gas Concentration (%)"=0.0, "Specific Arguments"="", "Comments"="", "Row No"=0, "Row Type Selector"=enum."Move Traverse Only", "Completion time"="", "Row Duration (mins)"=0.0, "No. of Valid pts."=0, "Meas Setup File"=""}, {"Start X"=0.0, "Start Y"=0.0, "Start Z"=805.0, "End X"=0.0, "End Y"=0.0, "End Z"=805.0, "No. of pts."=0, "Spacing"=enum."Linear", "Filename"=path "", "Tunnel Speed"=7.64, "Averaging time (min)"=0.0, "Extra Commands"="!Work in Tunnel Coordinates", "Carrier_1 Q (l/min)"=0.0, "Carrier_2 Q (l/min)"=0.0, "Trace Gas Concentration (%)"=0.0, "Specific Arguments"="MoveTT.vi;270", "Comments"="", "Row No"=0, "Row Type Selector"=enum."Run VI Named:", "Completion time"="", "Row Duration (mins)"=0.0, "No. of Valid pts."=0, "Meas Setup File"=""}, {"Start X"=-72.9, "Start Y"=-56.5, "Start Z"=12.7, "End X"=-72.9, "End Y"=-56.5, "End Z"=25.4, "No. of pts."=3, "Spacing"=enum."Specified", "Filename"=path "M:/\\Projects\\8773\\Results\\Tunnel1\\AnemometerSurvey.xls", "Tunnel Speed"=7.64, "Averaging time (min)"=1.0, "Extra Commands"="", "Carrier_1 Q (l/min)"=0.0, "Carrier_2 Q (l/min)"=0.0, "Trace Gas Concentration (%)"=0.0, "Specific Arguments"="Z= ;12.7;19.1;25.4\r", "Comments"="Anemo1", "Row No"=0, "Row Type Selector"=enum."Vertical Profile", "Completion time"="", "Row Duration (mins)"=0.0, "No. of Valid pts."=0, "Meas Setup File"="Current_Setup.xls"}, {"Start X"=-458.4, "Start Y"=87.9, "Start Z"=25.6, "End X"=-458.4, "End Y"=87.9, "End Z"=38.3, "No. of pts."=3, "Spacing"=enum."Specified", "Filename"=path "M:/\\Projects\\8773\\Results\\Tunnel1\\AnemometerSurvey.xls", "Tunnel Speed"=7.64, "Averaging time (min)"=1.0, "Extra Commands"="", "Carrier_1 Q (l/min)"=0.0, "Carrier_2 Q (l/min)"=0.0, "Trace Gas Concentration (%)"=0.0, "Specific Arguments"="Z= ;25.6;32.0;38.3\r", "Comments"="Anemo2", "Row No"=0, "Row Type Selector"=enum."Vertical Profile", "Completion time"="", "Row Duration (mins)"=0.0, "No. of Valid pts."=0, "Meas Setup File"="Current_Setup.xls"}, {"Start X"=0.0, "Start Y"=0.0, "Start Z"=150.0, "End X"=0.0, "End Y"=0.0, "End Z"=150.0, "No. of pts."=0, "Spacing"=enum."Linear", "Filename"=path "", "Tunnel Speed"=7.64, "Averaging time (min)"=0.0, "Extra Commands"="!Work in Tunnel Coordinates", "Carrier_1 Q (l/min)"=0.0, "Carrier_2 Q (l/min)"=0.0, "Trace Gas Concentration (%)"=0.0, "Specific Arguments"="", "Comments"="", "Row No"=0, "Row Type Selector"=enum."Move Traverse Only", "Completion time"="", "Row Duration (mins)"=0.0, "No. of Valid pts."=0, "Meas Setup File"=""}, {"Start X"=0.0, "Start Y"=0.0, "Start Z"=805.0, "End X"=0.0, "End Y"=0.0, "End Z"=805.0, "No. of pts."=0, "Spacing"=enum."Linear", "Filename"=path "", "Tunnel Speed"=7.64, "Averaging time (min)"=0.0, "Extra Commands"="!Work in Tunnel Coordinates", "Carrier_1 Q (l/min)"=0.0, "Carrier_2 Q (l/min)"=0.0, "Trace Gas Concentration (%)"=0.0, "Specific Arguments"="MoveTT.vi;290", "Comments"="", "Row No"=0, "Row Type Selector"=enum."Run VI Named:", "Completion time"="", "Row Duration (mins)"=0.0, "No. of Valid pts."=0, "Meas Setup File"=""}, {"Start X"=-72.9, "Start Y"=-56.5, "Start Z"=12.7, "End X"=-72.9, "End Y"=-56.5, "End Z"=25.4, "No. of pts."=3, "Spacing"=enum."Specified", "Filename"=path "M:/\\Projects\\8773\\Results\\Tunnel1\\AnemometerSurvey.xls", "Tunnel Speed"=7.64, "Averaging time (min)"=1.0, "Extra Commands"="", "Carrier_1 Q (l/min)"=0.0, "Carrier_2 Q (l/min)"=0.0, "Trace Gas Concentration (%)"=0.0, "Specific Arguments"="Z= ;12.7;19.1;25.4\r", "Comments"="Anemo1", "Row No"=0, "Row Type Selector"=enum."Vertical Profile", "Completion time"="", "Row Duration (mins)"=0.0, "No. of Valid pts."=0, "Meas Setup File"="Current_Setup.xls"}, {"Start X"=-458.4, "Start Y"=87.9, "Start Z"=25.6, "End X"=-458.4, "End Y"=87.9, "End Z"=38.3, "No. of pts."=3, "Spacing"=enum."Specified", "Filename"=path "M:/\\Projects\\8773\\Results\\Tunnel1\\AnemometerSurvey.xls", "Tunnel Speed"=7.64, "Averaging time (min)"=1.0, "Extra Commands"="", "Carrier_1 Q (l/min)"=0.0, "Carrier_2 Q (l/min)"=0.0, "Trace Gas Concentration (%)"=0.0, "Specific Arguments"="Z= ;25.6;32.0;38.3\r", "Comments"="Anemo2", "Row No"=0, "Row Type Selector"=enum."Vertical Profile", "Completion time"="", "Row Duration (mins)"=0.0, "No. of Valid pts."=0, "Meas Setup File"="Current_Setup.xls"}, {"Start X"=0.0, "Start Y"=0.0, "Start Z"=150.0, "End X"=0.0, "End Y"=0.0, "End Z"=150.0, "No. of pts."=0, "Spacing"=enum."Linear", "Filename"=path "", "Tunnel Speed"=7.64, "Averaging time (min)"=0.0, "Extra Commands"="!Work in Tunnel Coordinates", "Carrier_1 Q (l/min)"=0.0, "Carrier_2 Q (l/min)"=0.0, "Trace Gas Concentration (%)"=0.0, "Specific Arguments"="", "Comments"="", "Row No"=0, "Row Type Selector"=enum."Move Traverse Only", "Completion time"="", "Row Duration (mins)"=0.0, "No. of Valid pts."=0, "Meas Setup File"=""}, {"Start X"=0.0, "Start Y"=0.0, "Start Z"=805.0, "End X"=0.0, "End Y"=0.0, "End Z"=805.0, "No. of pts."=0, "Spacing"=enum."Linear", "Filename"=path "", "Tunnel Speed"=7.64, "Averaging time (min)"=0.0, "Extra Commands"="!Work in Tunnel Coordinates", "Carrier_1 Q (l/min)"=0.0, "Carrier_2 Q (l/min)"=0.0, "Trace Gas Concentration (%)"=0.0, "Specific Arguments"="MoveTT.vi;310", "Comments"="", "Row No"=0, "Row Type Selector"=enum."Run VI Named:", "Completion time"="", "Row Duration (mins)"=0.0, "No. of Valid pts."=0, "Meas Setup File"=""}, {"Start X"=-72.9, "Start Y"=-56.5, "Start Z"=12.7, "End X"=-72.9, "End Y"=-56.5, "End Z"=25.4, "No. of pts."=3, "Spacing"=enum."Specified", "Filename"=path "M:/\\Projects\\8773\\Results\\Tunnel1\\AnemometerSurvey.xls", "Tunnel Speed"=7.64, "Averaging time (min)"=1.0, "Extra Commands"="", "Carrier_1 Q (l/min)"=0.0, "Carrier_2 Q (l/min)"=0.0, "Trace Gas Concentration (%)"=0.0, "Specific Arguments"="Z= ;12.7;19.1;25.4\r", "Comments"="Anemo1", "Row No"=0, "Row Type Selector"=enum."Vertical Profile", "Completion time"="", "Row Duration (mins)"=0.0, "No. of Valid pts."=0, "Meas Setup File"="Current_Setup.xls"}, {"Start X"=-458.4, "Start Y"=87.9, "Start Z"=25.6, "End X"=-458.4, "End Y"=87.9, "End Z"=38.3, "No. of pts."=3, "Spacing"=enum."Specified", "Filename"=path "M:/\\Projects\\8773\\Results\\Tunnel1\\AnemometerSurvey.xls", "Tunnel Speed"=7.64, "Averaging time (min)"=1.0, "Extra Commands"="", "Carrier_1 Q (l/min)"=0.0, "Carrier_2 Q (l/min)"=0.0, "Trace Gas Concentration (%)"=0.0, "Specific Arguments"="Z= ;25.6;32.0;38.3\r", "Comments"="Anemo2", "Row No"=0, "Row Type Selector"=enum."Vertical Profile", "Completion time"="", "Row Duration (mins)"=0.0, "No. of Valid pts."=0, "Meas Setup File"="Current_Setup.xls"}, {"Start X"=0.0, "Start Y"=0.0, "Start Z"=150.0, "End X"=0.0, "End Y"=0.0, "End Z"=150.0, "No. of pts."=0, "Spacing"=enum."Linear", "Filename"=path "", "Tunnel Speed"=7.64, "Averaging time (min)"=0.0, "Extra Commands"="!Work in Tunnel Coordinates", "Carrier_1 Q (l/min)"=0.0, "Carrier_2 Q (l/min)"=0.0, "Trace Gas Concentration (%)"=0.0, "Specific Arguments"="", "Comments"="", "Row No"=0, "Row Type Selector"=enum."Move Traverse Only", "Completion time"="", "Row Duration (mins)"=0.0, "No. of Valid pts."=0, "Meas Setup File"=""}, {"Start X"=0.0, "Start Y"=0.0, "Start Z"=805.0, "End X"=0.0, "End Y"=0.0, "End Z"=805.0, "No. of pts."=0, "Spacing"=enum."Linear", "Filename"=path "", "Tunnel Speed"=7.64, "Averaging time (min)"=0.0, "Extra Commands"="!Work in Tunnel Coordinates", "Carrier_1 Q (l/min)"=0.0, "Carrier_2 Q (l/min)"=0.0, "Trace Gas Concentration (%)"=0.0, "Specific Arguments"="MoveTT.vi;330", "Comments"="", "Row No"=0, "Row Type Selector"=enum."Run VI Named:", "Completion time"="", "Row Duration (mins)"=0.0, "No. of Valid pts."=0, "Meas Setup File"=""}, {"Start X"=-72.9, "Start Y"=-56.5, "Start Z"=12.7, "End X"=-72.9, "End Y"=-56.5, "End Z"=25.4, "No. of pts."=3, "Spacing"=enum."Specified", "Filename"=path "M:/\\Projects\\8773\\Results\\Tunnel1\\AnemometerSurvey.xls", "Tunnel Speed"=7.64, "Averaging time (min)"=1.0, "Extra Commands"="", "Carrier_1 Q (l/min)"=0.0, "Carrier_2 Q (l/min)"=0.0, "Trace Gas Concentration (%)"=0.0, "Specific Arguments"="Z= ;12.7;19.1;25.4\r", "Comments"="Anemo1", "Row No"=0, "Row Type Selector"=enum."Vertical Profile", "Completion time"="", "Row Duration (mins)"=0.0, "No. of Valid pts."=0, "Meas Setup File"="Current_Setup.xls"}, {"Start X"=-458.4, "Start Y"=87.9, "Start Z"=25.6, "End X"=-458.4, "End Y"=87.9, "End Z"=38.3, "No. of pts."=3, "Spacing"=enum."Specified", "Filename"=path "M:/\\Projects\\8773\\Results\\Tunnel1\\AnemometerSurvey.xls", "Tunnel Speed"=7.64, "Averaging time (min)"=1.0, "Extra Commands"="", "Carrier_1 Q (l/min)"=0.0, "Carrier_2 Q (l/min)"=0.0, "Trace Gas Concentration (%)"=0.0, "Specific Arguments"="Z= ;25.6;32.0;38.3\r", "Comments"="Anemo2", "Row No"=0, "Row Type Selector"=enum."Vertical Profile", "Completion time"="", "Row Duration (mins)"=0.0, "No. of Valid pts."=0, "Meas Setup File"="Current_Setup.xls"}, {"Start X"=0.0, "Start Y"=0.0, "Start Z"=150.0, "End X"=0.0, "End Y"=0.0, "End Z"=150.0, "No. of pts."=0, "Spacing"=enum."Linear", "Filename"=path "", "Tunnel Speed"=7.64, "Averaging time (min)"=0.0, "Extra Commands"="!Work in Tunnel Coordinates", "Carrier_1 Q (l/min)"=0.0, "Carrier_2 Q (l/min)"=0.0, "Trace Gas Concentration (%)"=0.0, "Specific Arguments"="", "Comments"="", "Row No"=0, "Row Type Selector"=enum."Move Traverse Only", "Completion time"="", "Row Duration (mins)"=0.0, "No. of Valid pts."=0, "Meas Setup File"=""}, {"Start X"=0.0, "Start Y"=0.0, "Start Z"=805.0, "End X"=0.0, "End Y"=0.0, "End Z"=805.0, "No. of pts."=0, "Spacing"=enum."Linear", "Filename"=path "", "Tunnel Speed"=7.64, "Averaging time (min)"=0.0, "Extra Commands"="!Work in Tunnel Coordinates", "Carrier_1 Q (l/min)"=0.0, "Carrier_2 Q (l/min)"=0.0, "Trace Gas Concentration (%)"=0.0, "Specific Arguments"="MoveTT.vi;350", "Comments"="", "Row No"=0, "Row Type Selector"=enum."Run VI Named:", "Completion time"="", "Row Duration (mins)"=0.0, "No. of Valid pts."=0, "Meas Setup File"=""}, {"Start X"=-72.9, "Start Y"=-56.5, "Start Z"=12.7, "End X"=-72.9, "End Y"=-56.5, "End Z"=25.4, "No. of pts."=3, "Spacing"=enum."Specified", "Filename"=path "M:/\\Projects\\8773\\Results\\Tunnel1\\AnemometerSurvey.xls", "Tunnel Speed"=7.64, "Averaging time (min)"=1.0, "Extra Commands"="", "Carrier_1 Q (l/min)"=0.0, "Carrier_2 Q (l/min)"=0.0, "Trace Gas Concentration (%)"=0.0, "Specific Arguments"="Z= ;12.7;19.1;25.4\r", "Comments"="Anemo1", "Row No"=0, "Row Type Selector"=enum."Vertical Profile", "Completion time"="", "Row Duration (mins)"=0.0, "No. of Valid pts."=0, "Meas Setup File"="Current_Setup.xls"}, {"Start X"=-458.4, "Start Y"=87.9, "Start Z"=25.6, "End X"=-458.4, "End Y"=87.9, "End Z"=38.3, "No. of pts."=3, "Spacing"=enum."Specified", "Filename"=path "M:/\\Projects\\8773\\Results\\Tunnel1\\AnemometerSurvey.xls", "Tunnel Speed"=7.64, "Averaging time (min)"=1.0, "Extra Commands"="", "Carrier_1 Q (l/min)"=0.0, "Carrier_2 Q (l/min)"=0.0, "Trace Gas Concentration (%)"=0.0, "Specific Arguments"="Z= ;25.6;32.0;38.3\r", "Comments"="Anemo2", "Row No"=0, "Row Type Selector"=enum."Vertical Profile", "Completion time"="", "Row Duration (mins)"=0.0, "No. of Valid pts."=0, "Meas Setup File"="Current_Setup.xls"}, {"Start X"=0.0, "Start Y"=0.0, "Start Z"=805.0, "End X"=0.0, "End Y"=0.0, "End Z"=805.0, "No. of pts."=0, "Spacing"=enum."Linear", "Filename"=path "", "Tunnel Speed"=7.64, "Averaging time (min)"=0.0, "Extra Commands"="!Work in Tunnel Coordinates", "Carrier_1 Q (l/min)"=0.0, "Carrier_2 Q (l/min)"=0.0, "Trace Gas Concentration (%)"=0.0, "Specific Arguments"="MoveTT.vi;0.000000", "Comments"="", "Row No"=0, "Row Type Selector"=enum."Run VI Named:", "Completion time"="", "Row Duration (mins)"=0.0, "No. of Valid pts."=0, "Meas Setup File"=""}, {"Start X"=-3390.0, "Start Y"=-113.0, "Start Z"=780.0, "End X"=-3390.0, "End Y"=-113.0, "End Z"=780.0, "No. of pts."=0, "Spacing"=enum."Linear", "Filename"=path "M:/\\Projects\\8773\\Results\\Tunnel1\\AnemometerSurvey.xls", "Tunnel Speed"=0.0, "Averaging time (min)"=1.0, "Extra Commands"="!Work in Tunnel Coordinates", "Carrier_1 Q (l/min)"=0.0, "Carrier_2 Q (l/min)"=0.0, "Trace Gas Concentration (%)"=0.0, "Specific Arguments"="", "Comments"="Zeroes", "Row No"=0, "Row Type Selector"=enum."Single Measurement", "Completion time"="", "Row Duration (mins)"=0.0, "No. of Valid pts."=0, "Meas Setup File"="Current_Setup.xls"}, {"Start X"=-3390.0, "Start Y"=-113.0, "Start Z"=780.0, "End X"=-3390.0, "End Y"=-113.0, "End Z"=780.0, "No. of pts."=0, "Spacing"=enum."Linear", "Filename"=path "M:/\\Projects\\8773\\Results\\Tunnel1\\AnemometerSurvey.xls", "Tunnel Speed"=7.64, "Averaging time (min)"=1.0, "Extra Commands"="!Work in Tunnel Coordinates", "Carrier_1 Q (l/min)"=0.0, "Carrier_2 Q (l/min)"=0.0, "Trace Gas Concentration (%)"=0.0, "Specific Arguments"="", "Comments"="CalCheck", "Row No"=0, "Row Type Selector"=enum."Single Measurement", "Completion time"="", "Row Duration (mins)"=0.0, "No. of Valid pts."=0, "Meas Setup File"="Current_Setup.xls"}, {"Start X"=0.0, "Start Y"=0.0, "Start Z"=805.0, "End X"=0.0, "End Y"=0.0, "End Z"=805.0, "No. of pts."=0, "Spacing"=enum."Linear", "Filename"=path "M:/\\Projects\\8773\\Results\\Tunnel1\\AnemometerSurvey.xls", "Tunnel Speed"=7.64, "Averaging time (min)"=1.0, "Extra Commands"="!Work in Tunnel Coordinates", "Carrier_1 Q (l/min)"=0.0, "Carrier_2 Q (l/min)"=0.0, "Trace Gas Concentration (%)"=0.0, "Specific Arguments"="", "Comments"="Local CalCheck", "Row No"=0, "Row Type Selector"=enum."Single Measurement", "Completion time"="", "Row Duration (mins)"=0.0, "No. of Valid pts."=0, "Meas Setup File"="Current_Setup.xls"}, {"Start X"=-3390.0, "Start Y"=-113.0, "Start Z"=780.0, "End X"=-3390.0, "End Y"=-113.0, "End Z"=780.0, "No. of pts."=0, "Spacing"=enum."Linear", "Filename"=path "", "Tunnel Speed"=0.0, "Averaging time (min)"=0.0, "Extra Commands"="", "Carrier_1 Q (l/min)"=0.0, "Carrier_2 Q (l/min)"=0.0, "Trace Gas Concentration (%)"=0.0, "Specific Arguments"="", "Comments"="Tunnel Off", "Row No"=0, "Row Type Selector"=enum."Set Tunnel Speed Only", "Completion time"="", "Row Duration (mins)"=0.0, "No. of Valid pts."=0, "Meas Setup File"=""}] {"Carrier_2 Q (l/min)" format="%#.2f"; "Row Duration (mins)" format="%#.1f"; "Row No" min=0; "Trace Gas Concentration (%)" min=0.0 format="%#_4f"; "Carrier_1 Q (l/min)" format="%#.2f"; "Tunnel Speed" format="%#.2f"; "Start X" format="%#.2f"; "Start Y" format="%#.2f"; "Start Z" format="%#.2f"; "End X" format="%#.2f"; "End Y" format="%#.2f"; "End Z" format="%#.2f"; "Averaging time (min)" min=0.0 format="%#.2f"}
  in  "Tab Control":T4(tab)
  in  "Jump Bad Positions":bool=TRUE
  in  "Work in TUNNEL Coordinates":bool=TRUE
  in  "Command File Path / Name":path=path "/CentralDataCache/Projects/9999/Commands/Post_Processing_Machine/AnemometerSurvey.xls"
  in  "Results File Path / Name":path=path "/CentralDataCache/Projects/9999/Results/Post_Processing_Machine/AnemometerSurvey.xls"
  in  "Setup:":string(combo)="Current_Setup.xls"
  in  "Tunnel Warmup (min)":dbl=10.0
  in  "Velocity (m/s)":dbl=7.64
  in  "Measure (seconds)":dbl=60.0
  out "Measure (mins)":dbl=1.0
  in  "Multirun Closure Tasks":T5={"Turn Table --> Zero"=TRUE, "AutoCal"=FALSE, "Zeroes"=TRUE, "Global Cal Checks"=TRUE, "Local Cal Checks"=TRUE, "Tunnel Off"=TRUE}
  in  "Task Selection":T6={"Tunnel Warm Up"=TRUE, "AutoCal"=FALSE, "Zeroes"=TRUE, "Turn Table Schedule"=TRUE, "Global Cal Checks"=TRUE, "Local Cal Checks"=TRUE, "Vertical Profile"=TRUE, "Lateral Profile"=FALSE, "Reinitialize Task Array"=TRUE, "Save Command File"=TRUE, "Longitudinal Profile"=FALSE}
  in  "SpeedSettings":dbl[](array[numeric])
  in  "SingleMeasurement.Coords":T7(array[cluster])
  in  "Zeroes":T8={"X"=-3390.0, "Y"=-113.0, "Z"=780.0, "Use Tunnel Coords?"=TRUE, "RepeatEveryXDeg"=120.0}
  in  "Local Calcheck":T9={"X"=0.0, "Y"=0.0, "Z"=805.0, "Use Tunnel Coords? Coords"=TRUE, "RepeatEveryXDeg"=60.0}
  in  "Global Calcheck":T8={"X"=-3390.0, "Y"=-113.0, "Z"=780.0, "Use Tunnel Coords?"=TRUE, "RepeatEveryXDeg"=120.0}
  in  "Calculate TT Array":bool=TRUE
  in  "Angle Increment":dbl=20.0
  in  "Ending Angle":dbl=340.0
  in  "Starting Angle":dbl
  in  "Azimuth Values":dbl[](array[numeric])=[0.0, 20.0, 40.0, 60.0, 80.0, 100.0, 120.0, 140.0, 160.0, 180.0, 200.0, 220.0, 240.0, 260.0, 280.0, 300.0, 320.0, 340.0]
  in  "Build-A-Block":cluster{"Row Type Selector":T10, "Index":dbl}[](array[cluster])
  in  "VertProf.NumPts":dbl
  in  "VertProf.Coords END":cluster{"Z0":dbl}[](array[cluster])=[{"Z0"=0.0}, {"Z0"=12.9}]
  in  "VertSpacing":T11(ring)=enum."Specified"
  in  "VertProf.Coords":T12(array[cluster])=[{"X"=-72.9, "Y"=-56.5, "Z0"=0.0, "Name"="Anemo1"}, {"X"=-458.4, "Y"=87.9, "Z0"=12.9, "Name"="Anemo2"}]
  in  "Vert.Z-Locations":dbl[](array[numeric])=[12.7, 19.05, 25.4]
  in  "VP.TTHeightCorrs":T13={"TT.Azimuths"=[0.0, 20.0, 40.0, 60.0, 80.0, 100.0, 120.0, 140.0, 160.0, 180.0, 200.0, 220.0, 240.0, 260.0, 280.0, 300.0, 320.0, 340.0], "Z.HeightCorrs"=[[-0.0, -0.0], [-0.5, -1.4000000000000057], [-1.0, -3.1000000000000085], [-0.5, -4.1000000000000085], [-0.7999999999999972, -4.900000000000006], [-0.8999999999999915, -5.6000000000000085], [-0.3999999999999915, -5.5], [0.10000000000000853, -5.1000000000000085], [0.10000000000000853, -4.700000000000003], [0.5, -3.9000000000000057], [0.6000000000000085, -2.700000000000003], [0.10000000000000853, -2.1000000000000085], [0.6000000000000085, -0.9000000000000057], [0.6000000000000085, 0.29999999999999716], [0.29999999999999716, 0.8999999999999915], [0.7999999999999972, 1.7999999999999972], [0.7000000000000028, 2.200000000000003], [-0.0, 1.2000000000000028]], "Use Height Corrections"=TRUE, "Height Survey Filepaths"=[path "/CentralDataCache/Projects/8773/Results/Tunnel1/Height Survey & Corrections/Zsurvey-Anemo1.xls", path "/CentralDataCache/Projects/8773/Results/Tunnel1/Height Survey & Corrections/Zsurvey-Anemo2.xls"], "Corrections from File"=TRUE}
  in  "Correction Channel Name":string="T1:Z:Corrections"
  in  "LatProf.NumPts":dbl
  in  "LatProf.Coords END":cluster{"Y0":dbl}[](array[cluster])=[{"Y0"=-500.0}, {"Y0"=-500.0}, {"Y0"=-500.0}]
  in  "LatProf.Coords":T14(array[cluster])=[{"X"=1900.0, "Y0"=-500.0, "Z"=229.0, "Name"="TTLE"}, {"X"=0.0, "Y0"=-500.0, "Z"=229.0, "Name"="TTC"}, {"X"=1475.0, "Y0"=-500.0, "Z"=229.0, "Name"="TTTE"}]
  in  "Lat.Y-Locations":dbl[](array[numeric])=[-500.0, -400.0, -300.0, -200.0, -100.0, 0.0, 100.0, 200.0, 300.0, 400.0, 500.0]
  in  "Lat.HeightCorrs":T15={"Yvalues"=[0.0, 10.0, 20.0, 30.0, 40.0, 50.0, 60.0, 70.0, 80.0, 90.0, 100.0, 110.0, 120.0, 130.0, 140.0, 150.0, 160.0, 170.0, 180.0, 190.0, 200.0, 210.0, 220.0, 230.0, 240.0, 250.0, 260.0, 270.0, 280.0, 290.0, 300.0, 310.0, 320.0, 330.0, 340.0, 350.0], "X.HeightCorrs"=[[0.0], [-0.4], [-0.4], [-0.1], [0.6], [1.1], [1.5], [1.6], [1.5], [1.1], [0.3], [0.0], [-0.3], [-0.3], [-0.4], [0.7], [0.9], [1.8], [2.4], [2.5], [2.5], [2.2], [1.3], [0.7], [0.4], [0.0], [0.0], [0.8], [1.1], [1.7], [2.4], [2.4], [2.3], [2.3], [1.2], [0.4]], "Use Height Corrections"=FALSE}
  in  "LatSpacing":T11(ring)=enum."Specified"
  in  "LongSpacing":T11(ring)=enum."Specified"
  in  "LongProf.NumPts":dbl
  in  "LongProf.Coords END":cluster{"X0":dbl}[](array[cluster])=[{"X0"=1900.0}, {"X0"=0.0}, {"X0"=1475.0}]
  in  "LongProf.Coords":T16(array[cluster])=[{"X0"=1900.0, "Y"=-500.0, "Z"=229.0, "Name"="Window"}, {"X0"=0.0, "Y"=0.0, "Z"=229.0, "Name"="MidSpan"}, {"X0"=1475.0, "Y"=500.0, "Z"=229.0, "Name"="Wall"}]
  in  "Long.X-Locations":dbl[](array[numeric])=[-500.0, -250.0, 0.0, 250.0, 500.0]
  in  "Long.HeightCorrs":T17={"XValues"=[0.0, 10.0, 20.0, 30.0, 40.0, 50.0, 60.0, 70.0, 80.0, 90.0, 100.0, 110.0, 120.0, 130.0, 140.0, 150.0, 160.0, 170.0, 180.0, 190.0, 200.0, 210.0, 220.0, 230.0, 240.0, 250.0, 260.0, 270.0, 280.0, 290.0, 300.0, 310.0, 320.0, 330.0, 340.0, 350.0], "Y.HeightCorrs"=[[0.0], [-0.4], [-0.4], [-0.1], [0.6], [1.1], [1.5], [1.6], [1.5], [1.1], [0.3], [0.0], [-0.3], [-0.3], [-0.4], [0.7], [0.9], [1.8], [2.4], [2.5], [2.5], [2.2], [1.3], [0.7], [0.4], [0.0], [0.0], [0.8], [1.1], [1.7], [2.4], [2.4], [2.3], [2.3], [1.2], [0.4]], "Use Height Corrections"=FALSE}
  in  "MoveTrav.Coords":T18(array[cluster])
  in  "MessagesArray":string[](array[string])
  out "Audit Array":string[](array[string])=["Initialize", "Build TT Array", "Warm Up", "Zeroes", "AutoCal", "GlobalCalCheck", "LocalCalCheck", "Turn Table Schedule", "Vertical Corrections", "Vertical Profile", "Vertical Corrections", "Vertical Profile", "Lateral Profile", "Longitudinal Profile", "Repeat?", "Zeroes", "AutoCal", "GlobalCalCheck", "LocalCalCheck", "Turn Table Schedule", "Vertical Corrections", "Vertical Profile", "Vertical Corrections", "Vertical Profile", "Lateral Profile", "Longitudinal Profile", "Repeat?", "Zeroes", "AutoCal", "GlobalCalCheck", "LocalCalCheck", "Turn Table Schedule", "Vertical Corrections", "Vertical Profile", "Vertical Corrections", "Vertical Profile", "Lateral Profile", "Longitudinal Profile", "Repeat?", "Zeroes", "AutoCal", "GlobalCalCheck", "LocalCalCheck", "Turn Table Schedule", "Vertical Corrections", "Vertical Profile", "Vertical Corrections", "Vertical Profile", "Lateral Profile", "Longitudinal Profile", "Repeat?", "Zeroes", "AutoCal", "GlobalCalCheck", "LocalCalCheck", "Turn Table Schedule", "Vertical Corrections", "Vertical Profile", "Vertical Corrections", "Vertical Profile", "Lateral Profile", "Longitudinal Profile", "Repeat?", "Zeroes", "AutoCal", "GlobalCalCheck", "LocalCalCheck", "Turn Table Schedule", "Vertical Corrections", "Vertical Profile", "Vertical Corrections", "Vertical Profile", "Lateral Profile", "Longitudinal Profile", "Repeat?", "Zeroes", "AutoCal", "GlobalCalCheck", "LocalCalCheck", "Turn Table Schedule", "Vertical Corrections", "Vertical Profile", "Vertical Corrections", "Vertical Profile", "Lateral Profile", "Longitudinal Profile", "Repeat?", "Zeroes", "AutoCal", "GlobalCalCheck", "LocalCalCheck", "Turn Table Schedule", "Vertical Corrections", "Vertical Profile", "Vertical Corrections", "Vertical Profile", "Lateral Profile", "Longitudinal Profile", "Repeat?", "Zeroes", "AutoCal", "GlobalCalCheck", "LocalCalCheck", "Turn Table Schedule", "Vertical Corrections", "Vertical Profile", "Vertical Corrections", "Vertical Profile", "Lateral Profile", "Longitudinal Profile", "Repeat?", "Zeroes", "AutoCal", "GlobalCalCheck", "LocalCalCheck", "Turn Table Schedule", "Vertical Corrections", "Vertical Profile", "Vertical Corrections", "Vertical Profile", "Lateral Profile", "Longitudinal Profile", "Repeat?", "Zeroes", "AutoCal", "GlobalCalCheck", "LocalCalCheck", "Turn Table Schedule", "Vertical Corrections", "Vertical Profile", "Vertical Corrections", "Vertical Profile", "Lateral Profile", "Longitudinal Profile", "Repeat?", "Zeroes", "AutoCal", "GlobalCalCheck", "LocalCalCheck", "Turn Table Schedule", "Vertical Corrections", "Vertical Profile", "Vertical Corrections", "Vertical Profile", "Lateral Profile", "Longitudinal Profile", "Repeat?", "Zeroes", "AutoCal", "GlobalCalCheck", "LocalCalCheck", "Turn Table Schedule", "Vertical Corrections", "Vertical Profile", "Vertical Corrections", "Vertical Profile", "Lateral Profile", "Longitudinal Profile", "Repeat?", "Zeroes", "AutoCal", "GlobalCalCheck", "LocalCalCheck", "Turn Table Schedule", "Vertical Corrections", "Vertical Profile", "Vertical Corrections", "Vertical Profile", "Lateral Profile", "Longitudinal Profile", "Repeat?", "Zeroes", "AutoCal", "GlobalCalCheck", "LocalCalCheck", "Turn Table Schedule", "Vertical Corrections", "Vertical Profile", "Vertical Corrections", "Vertical Profile", "Lateral Profile", "Longitudinal Profile", "Repeat?", "Zeroes", "AutoCal", "GlobalCalCheck", "LocalCalCheck", "Turn Table Schedule", "Vertical Corrections", "Vertical Profile", "Vertical Corrections", "Vertical Profile", "Lateral Profile", "Longitudinal Profile", "Repeat?", "Zeroes", "AutoCal", "GlobalCalCheck", "LocalCalCheck", "Turn Table Schedule", "Vertical Corrections", "Vertical Profile", "Vertical Corrections", "Vertical Profile", "Lateral Profile", "Longitudinal Profile", "Repeat?", "Zeroes", "AutoCal", "GlobalCalCheck", "LocalCalCheck", "Turn Table Schedule", "Vertical Corrections", "Vertical Profile", "Vertical Corrections", "Vertical Profile", "Lateral Profile", "Longitudinal Profile", "Repeat?", "End"]
  in  "Index Tracking":T19
  in  "Stop Button":bool
  in  "RowTemplate":T20 {"Carrier_2 Q (l/min)" format="%#.2f"; "Row Duration (mins)" format="%#.1f"; "Row No" min=0; "Trace Gas Concentration (%)" min=0.0 format="%#_4f"; "Carrier_1 Q (l/min)" format="%#.2f"; "Tunnel Speed" format="%#.2f"; "Start X" format="%#.2f"; "Start Y" format="%#.2f"; "Start Z" format="%#.2f"; "End X" format="%#.2f"; "End Y" format="%#.2f"; "End Z" format="%#.2f"; "Averaging time (min)" min=0.0 format="%#.2f"}
  # "X           Y            Z"
  # "Start"
  # "End"
  # "X           Y            Z"
  # "Start"
  # "End"
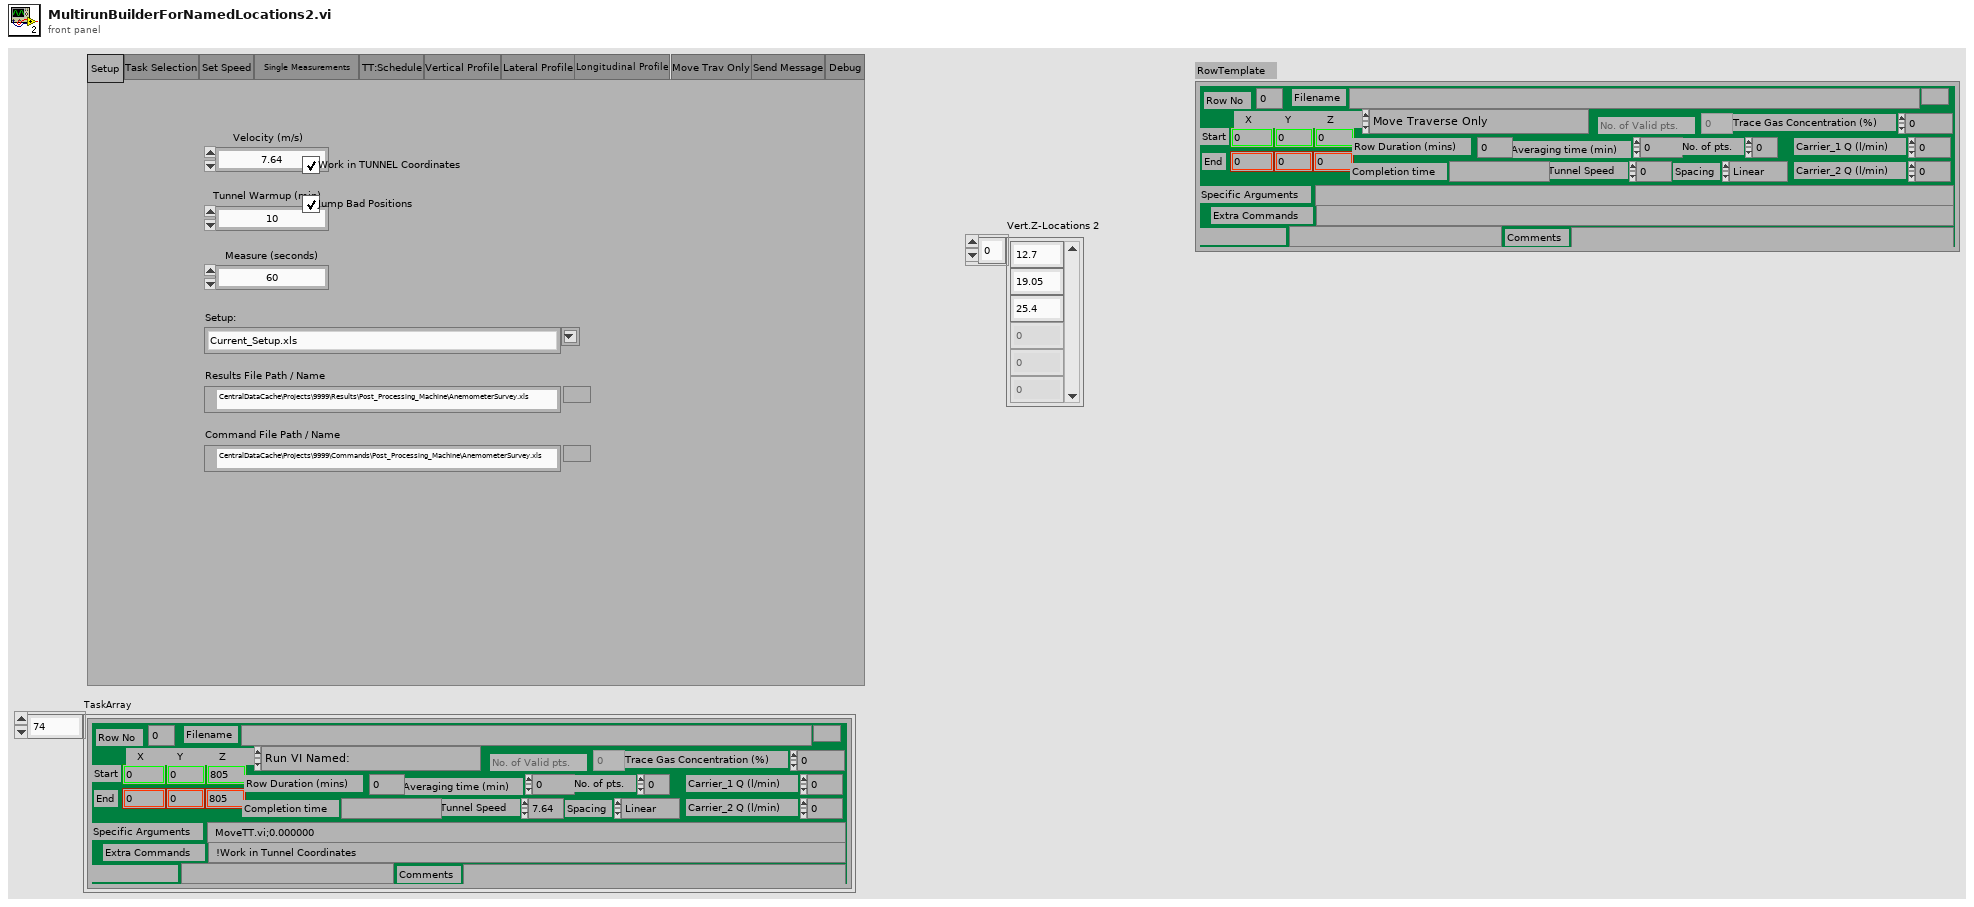
[diagram p1: front panel]
types:
  T1 = typedef "Spacing.ctl" = enum16{"Linear", "Log", "Gauss", "Specified", "N/A"}
  T2 = typedef "Multi_run_mode.ctl" = enum16{"Move Traverse Only", "Set Tunnel Speed Only", "Set Source Only", "Set Measurement Conditions", "Single Measurement", "Vertical Profile", "Lateral Profile", "Longitudinal Profile", "Explore Volume", "Multi-Axis Profile", "Auto Calibrate", "Meas Fast FID Bkgnd", "Check Beam Power", "Scanning Valve Measurement", "Run VI Named:", "Set ADAM Ch", "Wait (minutes)", "Send Message", "Synchronize With:", "Fall Back to this Row", "Turn Off Row Repeating", "Blank Row", "Traverse 3D Volume"}
  T3 = cluster{"Start X":sgl, "Start Y":sgl, "Start Z":sgl, "End X":sgl, "End Y":sgl, "End Z":sgl, "No. of pts.":i32, "Spacing":T1, "Filename":path, "Tunnel Speed":dbl, "Averaging time (min)":dbl, "Extra Commands":string, "Carrier_1 Q (l/min)":dbl, "Carrier_2 Q (l/min)":dbl, "Trace Gas Concentration (%)":dbl, "Specific Arguments":string, "Comments":string, "Row No":i32, "Row Type Selector":T2, "Completion time":string, "Row Duration (mins)":dbl, "No. of Valid pts.":i32, "Meas Setup File":string}[]
  T4 = enum32{"Setup", "Task Selection", "Set Speed", "Single Measurements", "TT:Schedule", "Vertical Profile", "Lateral Profile", "Longitudinal Profile", "Move Trav Only", "Send Message", "Debug"}
  T5 = cluster{"Turn Table --> Zero":bool, "AutoCal":bool, "Zeroes":bool, "Global Cal Checks":bool, "Local Cal Checks":bool, "Tunnel Off":bool}
  T6 = cluster{"Tunnel Warm Up":bool, "AutoCal":bool, "Zeroes":bool, "Turn Table Schedule":bool, "Global Cal Checks":bool, "Local Cal Checks":bool, "Vertical Profile":bool, "Lateral Profile":bool, "Reinitialize Task Array":bool, "Save Command File":bool, "Longitudinal Profile":bool}
  T7 = cluster{"X":dbl, "Y":dbl, "Z":dbl, "Name":string, "Use Tunnel Coords?":bool}[]
  T8 = cluster{"X":dbl, "Y":dbl, "Z":dbl, "Use Tunnel Coords?":bool, "RepeatEveryXDeg":dbl}
  T9 = cluster{"X":dbl, "Y":dbl, "Z":dbl, "Use Tunnel Coords? Coords":bool, "RepeatEveryXDeg":dbl}
  T10 = typedef "MRBRowTaskSelector.ctl" = enum16{"Move Traverse Only", "Set Tunnel Speed Only", "Set Source Only", "Set Measurement Conditions", "Single Measurement", "Vertical Profile", "Lateral Profile", "Longitudinal Profile", "Explore Volume", "Multi-Axis Profile", "Auto Calibrate", "Meas Fast FID Bkgnd", "Check Beam Power", "Scanning Valve Measurement", "Run VI Named:", "MoveTT", "TravZSurvey", "Set ADAM Ch", "Wait (minutes)", "Send Message", "Synchronize With:", "Fall Back to this Row", "Turn Off Row Repeating", "Blank Row", "Traverse 3D Volume"}
  T11 = enum16{"Linear", "Log", "Gauss", "Specified", "N/A"}
  T12 = cluster{"X":dbl, "Y":dbl, "Z0":dbl, "Name":string}[]
  T13 = cluster{"TT.Azimuths":dbl[], "Z.HeightCorrs":dbl[][], "Use Height Corrections":bool, "Height Survey Filepaths":path[], "Corrections from File":bool}
  T14 = cluster{"X":dbl, "Y0":dbl, "Z":dbl, "Name":string}[]
  T15 = cluster{"Yvalues":dbl[], "X.HeightCorrs":dbl[][], "Use Height Corrections":bool}
  T16 = cluster{"X0":dbl, "Y":dbl, "Z":dbl, "Name":string}[]
  T17 = cluster{"XValues":dbl[], "Y.HeightCorrs":dbl[][], "Use Height Corrections":bool}
  T18 = cluster{"X":dbl, "Y":dbl, "Z":dbl, "Use Tunnel Coords?":bool}[]
  T19 = cluster{"Azimuth Array Index":u32, "Vert Prof Array Index":u32, "Lat Prof Array Index":u32, "Long Prof Array Index":u32}
  T20 = cluster{"Start X":sgl, "Start Y":sgl, "Start Z":sgl, "End X":sgl, "End Y":sgl, "End Z":sgl, "No. of pts.":i32, "Spacing":T1, "Filename":path, "Tunnel Speed":dbl, "Averaging time (min)":dbl, "Extra Commands":string, "Carrier_1 Q (l/min)":dbl, "Carrier_2 Q (l/min)":dbl, "Trace Gas Concentration (%)":dbl, "Specific Arguments":string, "Comments":string, "Row No":i32, "Row Type Selector":T2, "Completion time":string, "Row Duration (mins)":dbl, "No. of Valid pts.":i32, "Meas Setup File":string}
  T21 = cluster{"Azimuth Array Index":u32, "Vert Prof Array Index":u32, "Lat Prof Array Index":u32, "Azimuth Array Index 2":u32}
  T22 = cluster{"X":dbl, "Y":dbl, "Z":dbl, string, "Use Tunnel Coords?":bool}
  T23 = enum16{"Load Command File", "Save Command File", "Check Multi Run Prog", "Check Multi Run Prog With Live Moves", "Run Multi Run Prog"}
  T24 = typedef "Tunnel_Coordinates.ctl" = enum16{"Work in Tunnel Coordinates", "Work in Model Coordinates"}
  T25 = typedef "Setup_Filetype.ctl" = enum16{"Measurement Setups", "Calibration Setups", "General", "Results File Plotter Setups", "Speed Calib Tweaks"}
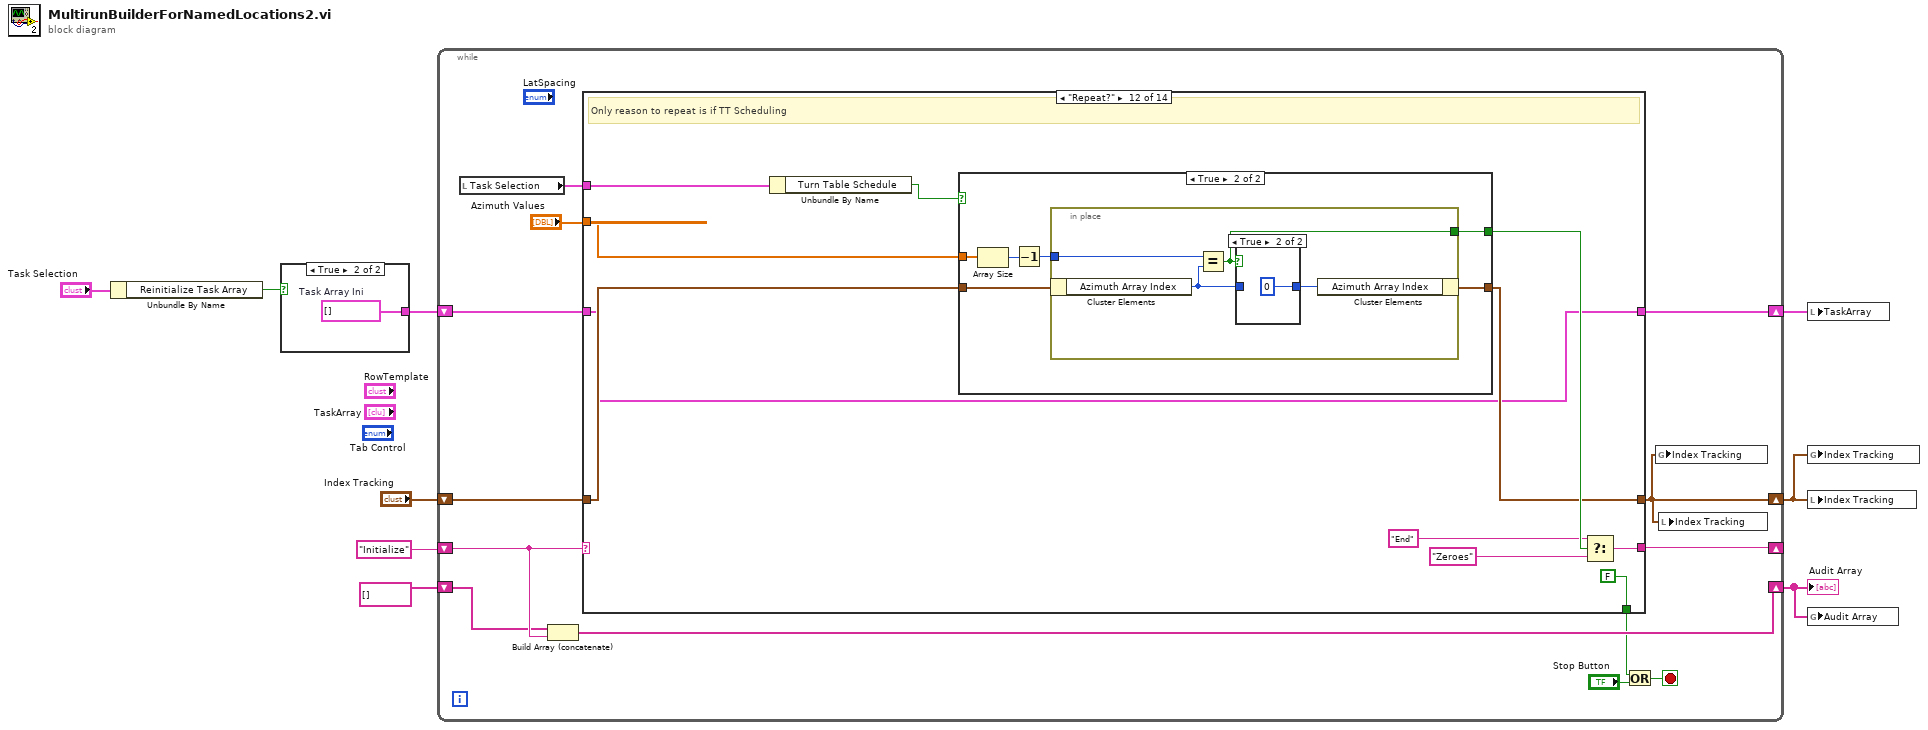
[diagram p0: block diagram]
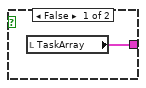
[diagram p2: hidden frame]
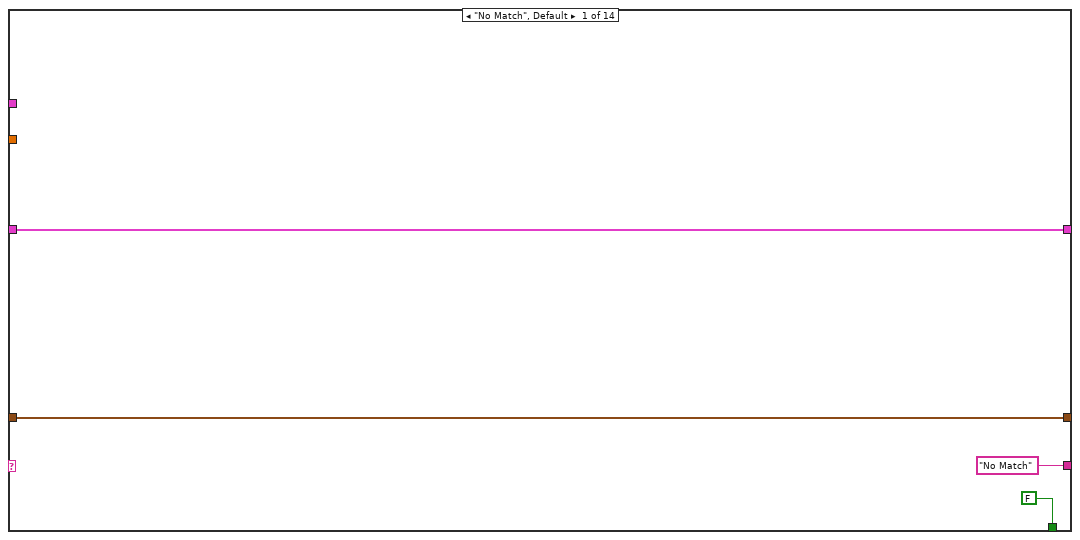
[diagram p3: hidden frame]
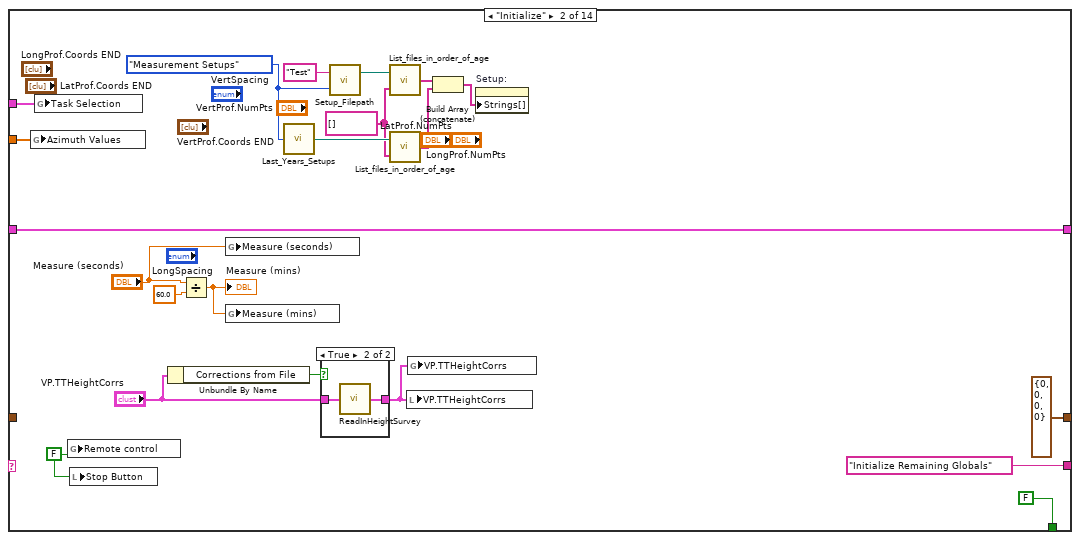
[diagram p4: hidden frame]
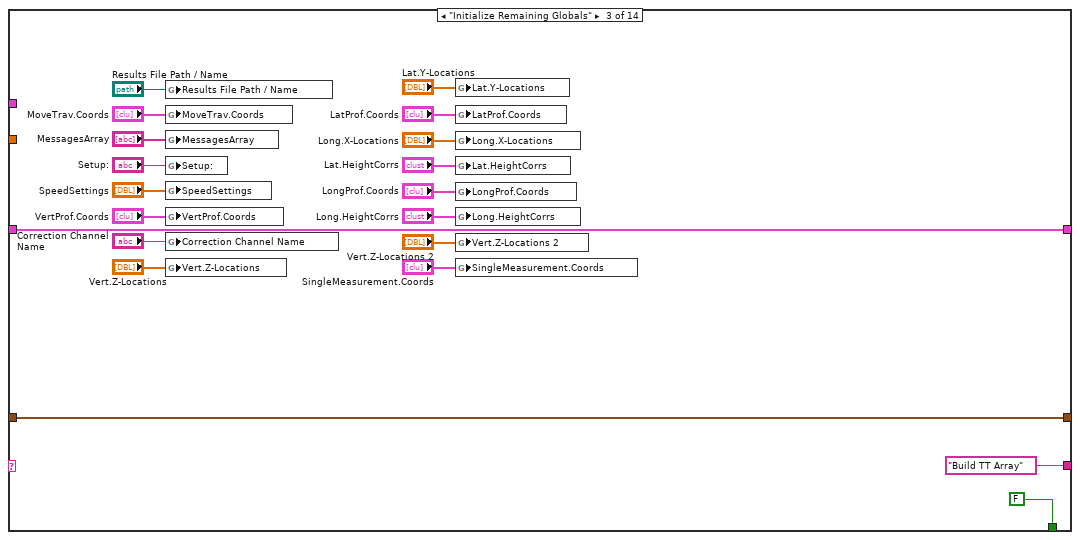
[diagram p6: hidden frame]
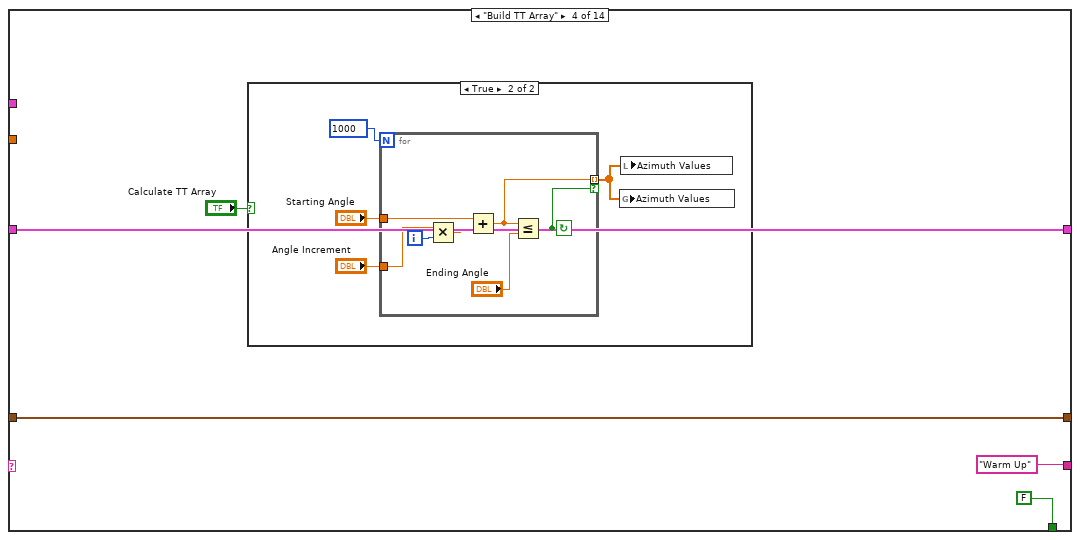
[diagram p7: hidden frame]
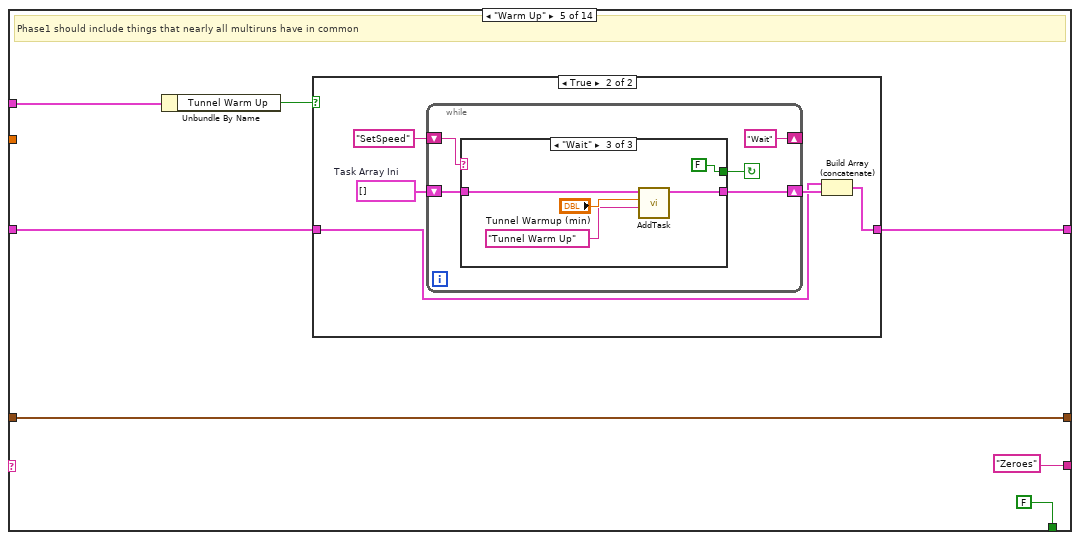
[diagram p9: hidden frame]
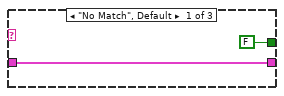
[diagram p11: hidden frame]
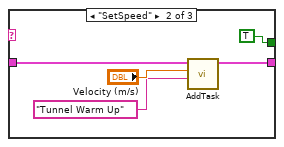
[diagram p12: hidden frame]
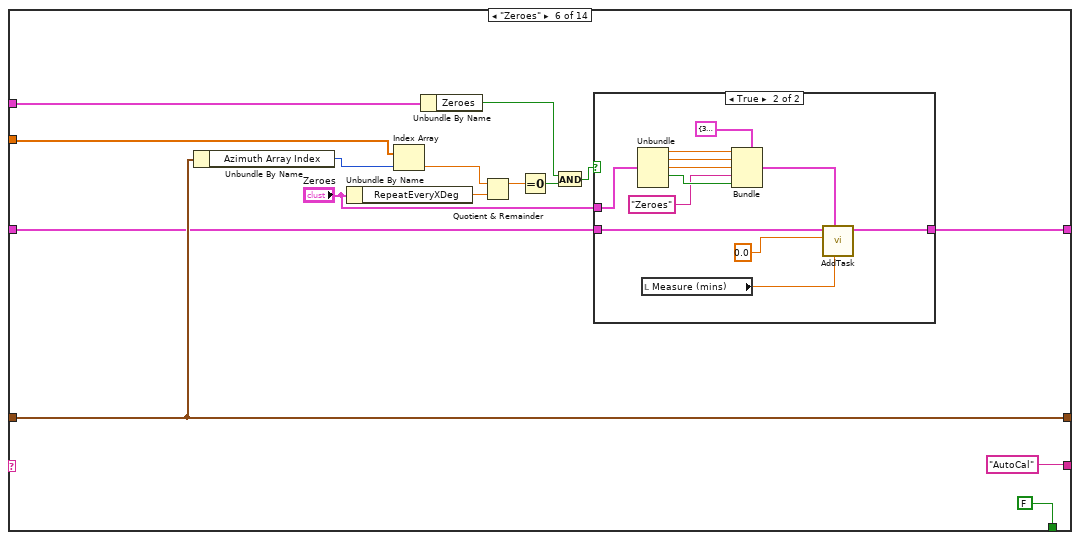
[diagram p13: hidden frame]
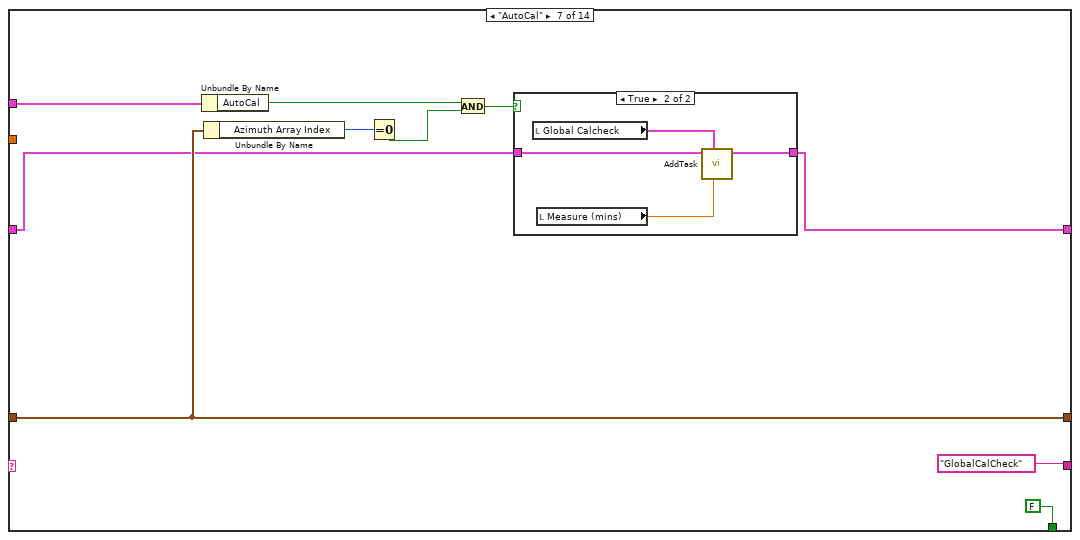
[diagram p15: hidden frame]
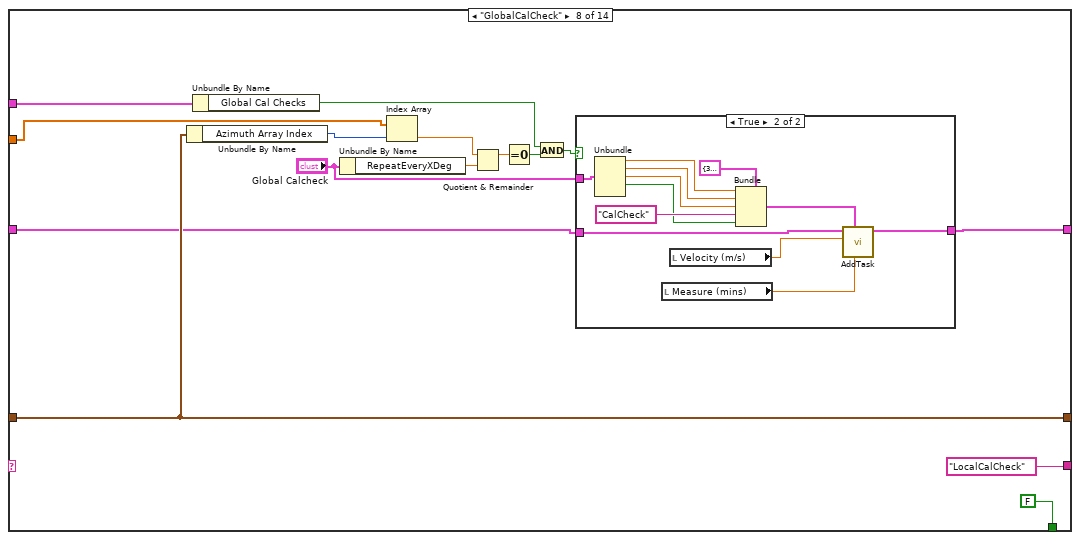
[diagram p17: hidden frame]
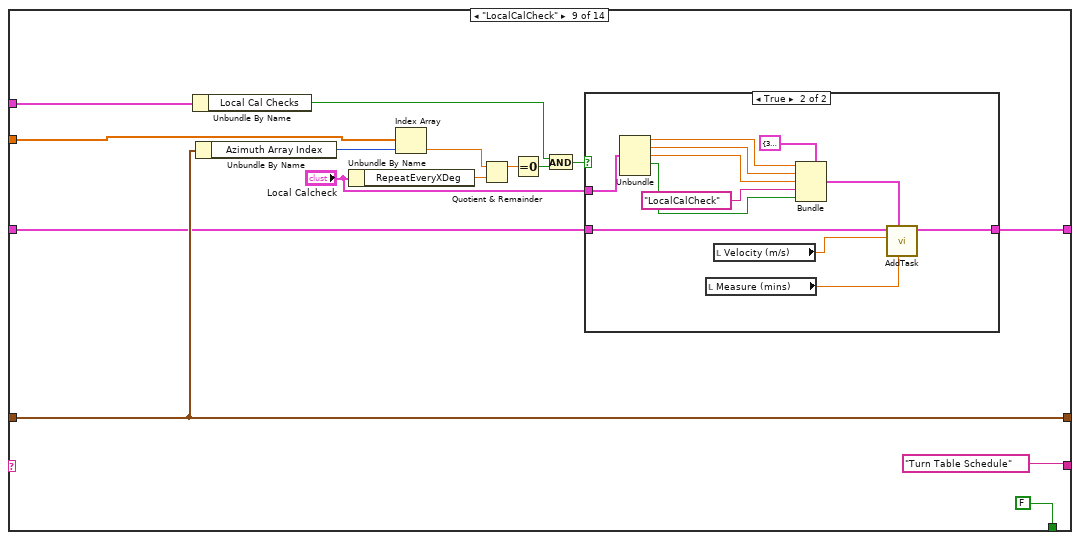
[diagram p19: hidden frame]
diagram:
  n1 = Unbundle By Name("Task Selection") -> ("Reinitialize Task Array"=w6:bool)
  n2 = case shown="True" w6 {
    tunnel: [w10 w11] -> w8
    frame False {
      n3 = local read "TaskArray"() -> (w10:T3)
    }
    frame True {
      w11 = T3 []  # Task Array Ini
    }
  }
  n4 = while {
    shift-right: [w24] -> _
    shift-left: "Initialize" -> [w22]
    shift-right: [w13] -> w1
    shift-left: w8 -> [w14]
    shift-right: [w21] -> w2
    shift-left: string[] [] -> [w20]
    shift-right: [w12] -> w3
    shift-left: "Index Tracking" -> [w23]
    stop <- w17 stop-if-true
    n5 = local read "Task Selection"() -> (w16:T6)
    n6 = Build Array (concatenate)(w20, w22) -> (w21:string[])
    n7 = case shown="\"Repeat?\"" w22 {
      tunnel: ["No Match" "Initialize Remaining Globals" "Build TT Array" "Warm Up" "Zeroes" "AutoCal" "GlobalCalCheck" "LocalCalCheck" "Turn Table Schedule" "Build-A-Block" "Repeat?" w244 "Save Multirun?" ("t") _] -> w24
      tunnel: [FALSE ("Stop Button") FALSE ("Stop Button") FALSE FALSE ("Stop Button") FALSE ("Stop Button") FALSE ("Stop Button") FALSE ("Stop Button") FALSE ("Stop Button") FALSE ("Stop Button") FALSE ("Stop Button") FALSE ("Stop Button") FALSE ("Stop Button") FALSE TRUE] -> w18
      tunnel: "Azimuth Values" -> [_ w35 _ _ _ w131 _ w165 w192 w224 _ w243 _ _]
      tunnel: w23 -> [w26 _ w55 w76 w93 w129 w153 w169 w198 w220 w234 w249 w277 w374]
      tunnel: [w26 T21 {"Azimuth Array Index"=0, "Vert Prof Array Index"=0, "Lat Prof Array Index"=0, "Azimuth Array Index 2"=0} ("Index Tracking") w55 w76 w93 w129 w153 w169 w198 w220 w234 w247 w277 w374] -> w12
      tunnel: w16 -> [_ w34 _ _ w92 w125 w149 w168 w197 w221 _ w240 _ w380]
      tunnel: w14 -> [w25 w36 w54 w73 w90 w119 w147 w162 w191 w219 w236 w241 w267 w377]
      tunnel: [w25 w36 w54 w73 w89 w120 w148 w163 w190 w218 w235 w241 w268 w376] -> w13
      frame "No Match", Default {
      }
      frame "Initialize" {
        w38 = FALSE ("Remote control")
        w48 = Setup_Filetype."Measurement Setups" ("Setup File Type")
        w43 = string[] [] ("file names")
        n8 = global write "MRCMDFBGlobal.vi" "Azimuth Values"(w35) -> ()
        n9 = global write "MRCMDFBGlobal.vi" "Task Selection"(w34) -> ()
        n10 = global write "Meas_global.vi" "Remote control"(w38) -> ()
        n11 = local write "Stop Button"(w38) -> ()
        n12 = Unbundle By Name("VP.TTHeightCorrs") -> ("Corrections from File"=w37:bool)
        n13 = Divide(x="Measure (seconds)", y=60.0 ("x")) -> (x/y=w33:dbl)
        "Measure (mins)" <- w33
        n14 = global write "MRCMDFBGlobal.vi" "Measure (seconds)"("Measure (seconds)") -> ()
        n15 = global write "MRCMDFBGlobal.vi" "Measure (mins)"(w33) -> ()
        n16 = call "Last_Years_Setups.vi"("Setup File Type"=w48) -> ("Directory"=w49:path)
        n17 = case shown="True" w37 {
          tunnel: "VP.TTHeightCorrs" -> [w50 w52]
          tunnel: [w50 w51] -> w30
          frame False {
          }
          frame True {
            n18 = call "ReadInHeightSurvey.vi"("VP.TTHeightCorrs In"=w52) -> ("VP.TTHeightCorrs Out"=w51:T13)
          }
        }
        n19 = call "Setup_Filepath.vi"("Setup File Type"=w48, "Filename in"="Test") -> ("Directory"=w47:path)  [unwired: 1 out]
        n20 = call "List_files_in_order_of_age.vi"("Files to Hide"=w43, "Folder"=w47) -> ("file names"=w46:string[])
        n21 = call "List_files_in_order_of_age.vi"("Files to Hide"=w43, "Folder"=w49) -> ("file names"=w45:string[])
        n22 = local write "VP.TTHeightCorrs"(w30) -> ()
        n23 = global write "MRCMDFBGlobal.vi" "VP.TTHeightCorrs"(w30) -> ()
        n24 = Build Array (concatenate)(w46, w45) -> (w42:string[])
        n25 = property on="Setup:" class="CmbBox"("Strings[]"=w42) -> ()  [unwired: 2 in, 2 out]
      }
      frame "Initialize Remaining Globals" {
        n26 = global write "MRCMDFBGlobal.vi" "Results File Path / Name"("Results File Path / Name") -> ()
        n27 = global write "MRCMDFBGlobal.vi" "MoveTrav.Coords"("MoveTrav.Coords") -> ()
        n28 = global write "MRCMDFBGlobal.vi" "MessagesArray"("MessagesArray") -> ()
        n29 = global write "MRCMDFBGlobal.vi" "Setup:"("Setup:") -> ()
        n30 = global write "MRCMDFBGlobal.vi" "SpeedSettings"("SpeedSettings") -> ()
        n31 = global write "MRCMDFBGlobal.vi" "VertProf.Coords"("VertProf.Coords") -> ()
        n32 = global write "MRCMDFBGlobal.vi" "Correction Channel Name"("Correction Channel Name") -> ()
        n33 = global write "MRCMDFBGlobal.vi" "Vert.Z-Locations"("Vert.Z-Locations") -> ()
        n34 = global write "MRCMDFBGlobal.vi" "Lat.Y-Locations"("Lat.Y-Locations") -> ()
        n35 = global write "MRCMDFBGlobal.vi" "LatProf.Coords"("LatProf.Coords") -> ()
        n36 = global write "MRCMDFBGlobal.vi" "Long.X-Locations"("Long.X-Locations") -> ()
        n37 = global write "MRCMDFBGlobal.vi" "Lat.HeightCorrs"("Lat.HeightCorrs") -> ()
        n38 = global write "MRCMDFBGlobal.vi" "LongProf.Coords"("LongProf.Coords") -> ()
        n39 = global write "MRCMDFBGlobal.vi" "Long.HeightCorrs"("Long.HeightCorrs") -> ()
        n40 = global write "MRCMDFBGlobal.vi" "Vert.Z-Locations 2"("Vert.Z-Locations 2") -> ()
        n41 = global write "MRCMDFBGlobal.vi" "SingleMeasurement.Coords"("SingleMeasurement.Coords") -> ()
      }
      frame "Build TT Array" {
        n42 = case shown="True" "Calculate TT Array" {
          frame False {
          }
          frame True {
            n43 = for {
              N: 1000 -> [_]
              tunnel: "Starting Angle" -> [w86]
              tunnel: "Angle Increment" -> [w87]
              tunnel: [w83] -> w78 mode=indexing if=w82
              i -> [w88]
              stop <- w82 continue-if-true
              n44 = Multiply(x=w87, y=w88) -> (x*y=w85:dbl)
              n45 = Add(x=w86, y=w85) -> (x+y=w83:dbl)
              n46 = Less Or Equal?(x=w83, y="Ending Angle") -> (x <= y?=w82:bool)
            }
            n47 = global write "MRCMDFBGlobal.vi" "Azimuth Values"(w78) -> ()
            n48 = local write "Azimuth Values"(w78) -> ()
          }
        }
      }
      frame "Warm Up" {
        # "Phase1 should include things that nearly all multiruns have in common"
        n49 = Unbundle By Name(w92) -> ("Tunnel Warm Up"=w91:bool)
        n50 = case shown="True" w91 {
          tunnel: w90 -> [w96 w98]
          tunnel: [w96 w97] -> w89
          frame False {
          }
          frame True {
            w100 = T3 []  # Task Array Ini
            n51 = while {
              shift-right: ["Wait"] -> _
              shift-left: "SetSpeed" -> [w106]
              shift-right: [w102] -> w99
              shift-left: w100 -> [w103]
              stop <- w104 continue-if-true
              n52 = case shown="\"Wait\"" w106 {
                tunnel: [FALSE TRUE FALSE] -> w104
                tunnel: w103 -> [w107 w110 w115]
                tunnel: [w107 w109 w114] -> w102
                frame "No Match", Default {
                }
                frame "SetSpeed" {
                  n53 = call-poly "AddTask.vi"("Comments"="Tunnel Warm Up", "Tunnel Speed"="Velocity (m/s)", "Input Task Array"=w110) -> ("Output Task Array"=w109:T3)  [unwired: 8 in]
                }
                frame "Wait" {
                  n54 = call-poly "AddTask.vi"("Comments"="Tunnel Warm Up", "Wait Time (min)"="Tunnel Warmup (min)", "Input Task Array"=w115) -> ("Output Task Array"=w114:T3)  [unwired: 8 in]
                }
              }
            }
            n55 = Build Array (concatenate)(w98, w99) -> (w97:T3)
          }
        }
      }
      frame "Zeroes" {
        n56 = Unbundle By Name(w129) -> ("Azimuth Array Index"=w130:u32)
        n57 = Unbundle By Name("Zeroes") -> ("RepeatEveryXDeg"=w127:dbl)
        n58 = Index Array(array=w131, index=w130) -> (element=w128:dbl)
        n59 = Unbundle By Name(w125) -> ("Zeroes"=w124:bool)
        n60 = Quotient & Remainder(x=w128, y=w127) -> (x-y*floor(x/y)=w126:dbl)  [unwired: 1 out]
        n61 = Equal To 0?(x=w126) -> (x = 0?=w123:bool)
        n62 = And(x=w124, y=w123) -> (x .and. y?=w122:bool)
        n63 = case shown="True" w122 {
          tunnel: "Zeroes" -> [_ w142]
          tunnel: [w134 w144] -> w120
          tunnel: w119 -> [w134 w143]
          frame False {
          }
          frame True {
            n64 = Unbundle(w142) -> ("X"=w140:dbl, "Y"=w139:dbl, "Z"=w138:dbl, "Use Tunnel Coords?"=w136:bool)  [unwired: 1 out]
            n65 = local read "Measure (mins)"() -> (w145:dbl)
            n66 = Bundle(cluster=T22 {"X"=36.0, "Y"=54.0, "Z"=300.0, "", "Use Tunnel Coords?"=TRUE} ("Coordinate Location"), "X"=w140, "Y"=w139, "Z"=w138, "Zeroes" ("Comments"), "Use Tunnel Coords?"=w136) -> (w137:T22)
            n67 = call-poly "AddTask.vi"("Averaging time (min)"=w145, "Coordinate Description"=w137, "Tunnel Speed"=0.0, "Input Task Array"=w143) -> ("Output Task Array"=w144:T3)  [unwired: 7 in]
          }
        }
      }
      frame "AutoCal" {
        n68 = Unbundle By Name(w149) -> ("AutoCal"=w151:bool)
        n69 = Unbundle By Name(w153) -> ("Azimuth Array Index"=w152:u32)
        n70 = Equal To 0?(x=w152) -> (x = 0?=w154:bool)
        n71 = And(x=w151, y=w154) -> (x .and. y?=w150:bool)
        n72 = case shown="True" w150 {
          tunnel: [w157 w159] -> w148
          tunnel: w147 -> [w157 w158]
          frame False {
          }
          frame True {
            n73 = local read "Global Calcheck"() -> (w160:T8)
            n74 = local read "Measure (mins)"() -> (w161:dbl)
            n75 = call-poly "AddTask.vi"("Averaging time (min)"=w161, "Global Calcheck"=w160, "Input Task Array"=w158) -> ("Output Task Array"=w159:T3)  [unwired: 8 in]
          }
        }
      }
      frame "GlobalCalCheck" {
        n76 = Unbundle By Name(w169) -> ("Azimuth Array Index"=w174:u32)
        n77 = Unbundle By Name(w168) -> ("Global Cal Checks"=w167:bool)
        n78 = Unbundle By Name("Global Calcheck") -> ("RepeatEveryXDeg"=w172:dbl)
        n79 = Index Array(array=w165, index=w174) -> (element=w173:dbl)
        n80 = Quotient & Remainder(x=w173, y=w172) -> (x-y*floor(x/y)=w171:dbl)  [unwired: 1 out]
        n81 = Equal To 0?(x=w171) -> (x = 0?=w170:bool)
        n82 = And(x=w167, y=w170) -> (x .and. y?=w164:bool)
        n83 = case shown="True" w164 {
          tunnel: "Global Calcheck" -> [_ w185]
          tunnel: [w177 w187] -> w163
          tunnel: w162 -> [w177 w186]
          frame False {
          }
          frame True {
            n84 = Unbundle(w185) -> ("X"=w182:dbl, "Y"=w181:dbl, "Z"=w180:dbl, "Use Tunnel Coords?"=w179:bool)  [unwired: 1 out]
            n85 = local read "Measure (mins)"() -> (w188:dbl)
            n86 = local read "Velocity (m/s)"() -> (w189:dbl)
            n87 = Bundle(cluster=T22 {"X"=36.0, "Y"=54.0, "Z"=300.0, "", "Use Tunnel Coords?"=TRUE} ("Coordinate Location"), "X"=w182, "Y"=w181, "Z"=w180, "CalCheck" ("Comments"), "Use Tunnel Coords?"=w179) -> (w178:T22)
            n88 = call-poly "AddTask.vi"("Averaging time (min)"=w188, "Coordinate Description"=w178, "Tunnel Speed"=w189, "Input Task Array"=w186) -> ("Output Task Array"=w187:T3)  [unwired: 7 in]
          }
        }
      }
      frame "LocalCalCheck" {
        n89 = Unbundle By Name(w197) -> ("Local Cal Checks"=w196:bool)
        n90 = Unbundle By Name(w198) -> ("Azimuth Array Index"=w202:u32)
        n91 = Unbundle By Name("Local Calcheck") -> ("RepeatEveryXDeg"=w200:dbl)
        n92 = Index Array(array=w192, index=w202) -> (element=w201:dbl)
        n93 = Quotient & Remainder(x=w201, y=w200) -> (x-y*floor(x/y)=w199:dbl)  [unwired: 1 out]
        n94 = Equal To 0?(x=w199) -> (x = 0?=w195:bool)
        n95 = And(x=w196, y=w195) -> (x .and. y?=w194:bool)
        n96 = case shown="True" w194 {
          tunnel: "Local Calcheck" -> [_ w213]
          tunnel: w191 -> [w205 w215]
          tunnel: [w205 w214] -> w190
          frame False {
          }
          frame True {
            n97 = Unbundle(w213) -> ("X"=w206:dbl, "Y"=w207:dbl, "Z"=w208:dbl, "Use Tunnel Coords? Coords"=w209:bool)  [unwired: 1 out]
            n98 = local read "Measure (mins)"() -> (w216:dbl)
            n99 = local read "Velocity (m/s)"() -> (w217:dbl)
            n100 = Bundle(cluster=T22 {"X"=36.0, "Y"=54.0, "Z"=300.0, "", "Use Tunnel Coords?"=TRUE} ("Coordinate Location"), "X"=w206, "Y"=w207, "Z"=w208, "LocalCalCheck" ("Comments"), "Use Tunnel Coords?"=w209) -> (w210:T22)
            n101 = call-poly "AddTask.vi"("Averaging time (min)"=w216, "Coordinate Description"=w210, "Tunnel Speed"=w217, "Input Task Array"=w215) -> ("Output Task Array"=w214:T3)  [unwired: 7 in]
          }
        }
      }
      frame "Turn Table Schedule" {
        n102 = Unbundle By Name(w221) -> ("Turn Table Schedule"=w222:bool)
        n103 = case shown="True" w222 {
          tunnel: w224 -> [_ w232]
          tunnel: w220 -> [_ w231]
          tunnel: w219 -> [w226 w230]
          tunnel: [w226 w229] -> w218
          frame False {
          }
          frame True {
            n104 = Unbundle By Name(w231) -> ("Azimuth Array Index"=w228:u32)
            n105 = Index Array(array=w232, index=w228) -> (element=w227:dbl)
            n106 = call-poly "AddTask.vi"("TT:Azimuth"=w227, "Input Task Array"=w230) -> ("Output Task Array"=w229:T3)  [unwired: 9 in]
          }
        }
      }
      frame "Build-A-Block" {
        n107 = call "MR_Build-A-Block.vi"("Build-A-Block"="Build-A-Block") -> ("TaskArray"=w237:T3)
        n108 = Build Array (concatenate)(w236, w237) -> (w235:T3)
      }
      frame "Repeat?" {
        # "Only reason to repeat is if TT Scheduling"
        n109 = Unbundle By Name(w240) -> ("Turn Table Schedule"=w242:bool)
        n110 = case shown="True" w242 {
          tunnel: w249 -> [w251 w258]
          tunnel: [TRUE w257] -> w248
          tunnel: [w251 w256] -> w247
          tunnel: w243 -> [_ w255]
          frame False {
          }
          frame True {
            n111 = Array Size(array=w255) -> (size(s)=w254:i32)
            n112 = Decrement(x=w254) -> (x-1=w253:i32)
            n113 = in-place {
              in-place-border: w253 -> [w260]
              in-place-border: [w261] -> w257
              n114 = in-place-cluster #1(w258) -> ("Azimuth Array Index"=w259:u32)
              n115 = Equal?(x=w260, y=w259) -> (x = y?=w261:bool)
              n116 = case shown="True" w261 {
                tunnel: [w263 0] -> w262
                tunnel: w259 -> [w264 _]
                frame False {
                  n117 = Increment(x=w264) -> (x+1=w263:u32)
                }
                frame True {
                }
              }
              n118 = in-place-cluster #1("Azimuth Array Index"=w262) -> (w256:T19)
            }
          }
        }
        n119 = Select(t="End", s=w248, f="Zeroes" ("t")) -> (s? t:f=w244:string)
      }
      frame "End" {
        n120 = Unbundle By Name("Multirun Closure Tasks") -> ("Turn Table --> Zero"=w274:bool, "Zeroes"=w273:bool, "AutoCal"=w272:bool, "Global Cal Checks"=w271:bool, "Local Cal Checks"=w270:bool, "Tunnel Off"=w269:bool)
        n121 = while {
          shift-right: [w288] -> _
          shift-left: "Turn Table" -> [w289]
          tunnel: w274 -> [w287]
          tunnel: w273 -> [w284]
          tunnel: w272 -> [w283]
          tunnel: w271 -> [w282]
          tunnel: w270 -> [w281]
          tunnel: w269 -> [w280]
          shift-right: [w285] -> w268
          shift-left: w267 -> [w286]
          stop <- w279 continue-if-true
          n122 = case shown="\"No Match\", Default" w289 {
            tunnel: [_ "Zeroes" "AutoCal" "GlobalCalCheck" "LocalCalCheck" "Tunnel Off" _] -> w288
            tunnel: w287 -> [_ w296 _ _ _ _ _]
            tunnel: w286 -> [w291 w295 w305 w323 w333 w351 w368]
            tunnel: [w291 w294 w304 w322 w332 w350 w367] -> w285
            tunnel: w284 -> [_ _ w301 _ _ _ _]
            tunnel: w283 -> [_ _ _ w319 _ _ _]
            tunnel: w282 -> [_ _ _ _ w330 _ _]
            tunnel: w281 -> [_ _ _ _ _ w348 _]
            tunnel: w280 -> [_ _ _ _ _ _ w366]
            tunnel: [FALSE TRUE TRUE TRUE TRUE TRUE TRUE] -> w279
            frame "No Match", Default {
            }
            frame "Turn Table" {
              n123 = case shown="True" w296 {
                tunnel: w295 -> [w297 w299]
                tunnel: [w297 w298] -> w294
                frame False {
                }
                frame True {
                  n124 = call-poly "AddTask.vi"("TT:Azimuth"=0.0, "Input Task Array"=w299) -> ("Output Task Array"=w298:T3)  [unwired: 9 in]
                }
              }
            }
            frame "Zeroes" {
              n125 = case shown="True" w301 {
                tunnel: w305 -> [w306 w317]
                tunnel: [w306 w316] -> w304
                frame False {
                }
                frame True {
                  n126 = local read "Zeroes"() -> (w314:T8)
                  n127 = Unbundle(w314) -> ("X"=w311:dbl, "Y"=w310:dbl, "Z"=w309:dbl, "Use Tunnel Coords?"=w308:bool)  [unwired: 1 out]
                  n128 = local read "Measure (mins)"() -> (w315:dbl)
                  n129 = Bundle(cluster=T22 {"X"=36.0, "Y"=54.0, "Z"=300.0, "", "Use Tunnel Coords?"=TRUE} ("Coordinate Location"), "X"=w311, "Y"=w310, "Z"=w309, "Zeroes" ("Comments"), "Use Tunnel Coords?"=w308) -> (w307:T22)
                  n130 = call-poly "AddTask.vi"("Averaging time (min)"=w315, "Coordinate Description"=w307, "Tunnel Speed"=0.0, "Input Task Array"=w317) -> ("Output Task Array"=w316:T3)  [unwired: 7 in]
                }
              }
            }
            frame "AutoCal" {
              n131 = case shown="True" w319 {
                tunnel: w323 -> [w324 w328]
                tunnel: [w324 w327] -> w322
                frame False {
                }
                frame True {
                  n132 = local read "Global Calcheck"() -> (w325:T8)
                  n133 = local read "Measure (mins)"() -> (w326:dbl)
                  n134 = call-poly "AddTask.vi"("Averaging time (min)"=w326, "Global Calcheck"=w325, "Input Task Array"=w328) -> ("Output Task Array"=w327:T3)  [unwired: 8 in]
                }
              }
            }
            frame "GlobalCalCheck" {
              n135 = case shown="True" w330 {
                tunnel: w333 -> [w334 w346]
                tunnel: [w334 w343] -> w332
                frame False {
                }
                frame True {
                  n136 = local read "Global Calcheck"() -> (w342:T8)
                  n137 = Unbundle(w342) -> ("X"=w338:dbl, "Y"=w337:dbl, "Z"=w336:dbl, "Use Tunnel Coords?"=w335:bool)  [unwired: 1 out]
                  n138 = local read "Measure (mins)"() -> (w344:dbl)
                  n139 = local read "Velocity (m/s)"() -> (w345:dbl)
                  n140 = Bundle(cluster=T22 {"X"=36.0, "Y"=54.0, "Z"=300.0, "", "Use Tunnel Coords?"=TRUE} ("Coordinate Location"), "X"=w338, "Y"=w337, "Z"=w336, "CalCheck" ("Comments"), "Use Tunnel Coords?"=w335) -> (w339:T22)
                  n141 = call-poly "AddTask.vi"("Averaging time (min)"=w344, "Coordinate Description"=w339, "Tunnel Speed"=w345, "Input Task Array"=w346) -> ("Output Task Array"=w343:T3)  [unwired: 7 in]
                }
              }
            }
            frame "LocalCalCheck" {
              n142 = case shown="True" w348 {
                tunnel: w351 -> [w352 w363]
                tunnel: [w352 w362] -> w350
                frame False {
                }
                frame True {
                  n143 = local read "Local Calcheck"() -> (w360:T9)
                  n144 = Unbundle(w360) -> ("X"=w358:dbl, "Y"=w357:dbl, "Z"=w356:dbl, "Use Tunnel Coords? Coords"=w353:bool)  [unwired: 1 out]
                  n145 = local read "Measure (mins)"() -> (w361:dbl)
                  n146 = local read "Velocity (m/s)"() -> (w364:dbl)
                  n147 = Bundle(cluster=T22 {"X"=36.0, "Y"=54.0, "Z"=300.0, "", "Use Tunnel Coords?"=TRUE} ("Coordinate Location"), "X"=w358, "Y"=w357, "Z"=w356, "LocalCalCheck" ("Comments"), "Use Tunnel Coords?"=w353) -> (w354:T22)
                  n148 = call-poly "AddTask.vi"("Averaging time (min)"=w361, "Coordinate Description"=w354, "Tunnel Speed"=w364, "Input Task Array"=w363) -> ("Output Task Array"=w362:T3)  [unwired: 7 in]
                }
              }
            }
            frame "Tunnel Off" {
              n149 = case shown="True" w366 {
                tunnel: w368 -> [w369 w371]
                tunnel: [w369 w370] -> w367
                frame False {
                }
                frame True {
                  n150 = call-poly "AddTask.vi"("Comments"="Tunnel Off", "Tunnel Speed"=0.0, "Input Task Array"=w371) -> ("Output Task Array"=w370:T3)  [unwired: 8 in]
                }
              }
            }
          }
        }
      }
      frame "Save Multirun?" {
        n151 = Unbundle By Name(w380) -> ("Save Command File"=w378:bool)
        n152 = case shown="True" w378 {
          tunnel: "Command File Path / Name" -> [_ w387]
          tunnel: w377 -> [w381 w382]
          tunnel: [w381 w382] -> w376
          frame False {
          }
          frame True {
            n153 = case shown="False" "Work in TUNNEL Coordinates" {
              tunnel: [Tunnel_Coordinates."Work in Model Coordinates" ("Work in Tunnel Coordinates?") Tunnel_Coordinates."Work in Tunnel Coordinates" ("Work in Tunnel Coordinates?")] -> w384
              frame False {
              }
              frame True {
              }
            }
            n154 = call "Multi_Run_Prog.vi"("Command filename"=w387, "Mode"=T23."Save Command File", "Table"=w382, "Work in Tunnel Coordinates?"=w384, "Jump Bad Positions"="Jump Bad Positions") -> ()  [unwired: 15 in]
          }
        }
      }
    }
    n155 = Or(x=w18, y="Stop Button") -> (x .or. y?=w17:bool)
    n156 = global write "MRCMDFBGlobal.vi" "Index Tracking"(w12) -> ()
    n157 = local write "Index Tracking"(w12) -> ()
  }
  "Audit Array" <- w2
  n158 = local write "TaskArray"(w1) -> ()
  n159 = global write "MRCMDFBGlobal.vi" "Index Tracking"(w3) -> ()
  n160 = local write "Index Tracking"(w3) -> ()
  n161 = global write "MRCMDFBGlobal.vi" "Audit Array"(w2) -> ()
